vi "CliftonStrengths.vi"() -> ()   [LabVIEW 2024]
uses:
  ctrl/ctrl_white_stringBox.ctl
  ctrl/ctrl_CB_talent.ctl
  ctrl/ctrl_CB_description.ctl
  ctrl/ctrl_enum_overview.ctl
  ctrl/ctrl_enum_adj.ctl
  <vilib>/Utility/miscctls.llb/LVPointTypeDef.ctl
panel:
  out "Talent2 CB":T1
  out "arr Description CB":string[](array[string])
  out "Talent order CB":string[](array[string])
  out "Description CB":T2
  out "Talent1 CB":T1
  out "Background CB":u32(colorbox)=16777226
  out "Background black CB":u32(colorbox)
  out "comp space":u32
  out "Theme compare":string[][](array[string])=[["1 가능성을 헤아리는 능력을 타고났습니다.", "3 현실을 헤아리는 능력을 타고났습니다."], ["1 다른 여러 경로를 고려합니다.", "25 단 하나의 목적지에 집중합니다."], ["2 관심이 가면 의지도 생깁니다.", "25 의지가 있어야 관심이 생깁니다."], ["2 항상 새로운 것을 배우는 데 관심이 있습니다.", "33 항상 새로운 사람을 만나는 데 관심이 있습니다."], ["3 머리를 따릅니다.", "5 가슴을 따릅니다."], ["3 진실은 객관적이며 측정할 수 있어야 합니다.", "16 진실은 정신적인 것이며 눈에 보이지 않을 수 있습니다."], ["4 성장과 배움을 위해 탐구하는 방식으로 접근함", "17 성장과 배움을 위해 습득하는 방식으로 접근함"], ["4 이해해야 할 개념에 대해 생각함", "34 해결해야 할 문제에 대해 생각함"], ["5 다른 사람의 기분을 잘 알아맞히는 편입니다.", "6 다른 사람의 성향을 잘 알아맞히는 편입니다."], ["5 직감에 따라 무엇을 해야 할지 결정합니다.", "3 데이터를 보고 무엇을 해야 할지 결정합니다."], ["6 당신이 누구인지 압니다.", "12 당신을 알고 싶고, 당신이 나를 알아주길 원합니다."], ["6 사람에서 출발해서 그 사람에게 적절한 일을 찾습니다.", "18 일에서 출발해서 그 일에 적절한 사람을 찾습니다."], ["7 제대로 못할 거라면 아예 시작도 하지 마십시오.", "20 아무것도 안 하는 것보다 뭐라도 하는 편이 낫습니다."], ["7 일을 제대로 하지 못하면 심한 죄책감이 듭니다.", "23 성공할 기회를 놓치면 너무나 후회가 됩니다."], ["8 적극적으로 개입하여 해결하기 위해 위험을 예측합니다.", "32 위험을 피하고 최소화하기 위해 위험을 예측합니다."], ["8 확신", "2 호기심"], ["9 외부에 있는 사람들을 수용하기 위해 노력합니다.", "28 내부에 있는 사람들의 합의를 도출하기 위해 노력합니다."], ["9 한 배에 탄 모든 사람을 차별없이 받아들입니다.", "10 배에 태울 사람을 선별적으로 선택합니다."], ["10 탁월함의 기준을 충족하거나 그 이상까지 달성하고 싶습니다.", "31 최고의 자리에 오르고 싶습니다."], ["10 훌륭한 성과를 쌓아가고 싶습니다.", "34 고장난 것을 고치고 싶습니다."], ["11 다른 사람들과 이야기할 때 생각이 잘 되고 가장 많이 배웁니다.", "4 혼자서 조용히 있을 때 생각이 잘 되고 가장 많이 배웁니다."], ["11 이야기를 하는 것은 사람들에게 나의 메시지를 이해시키는 데 도움이 됩니다.", "21 역사를 다시 이야기하는 것은 사람들이 과거를 기억하는 데 도움이 됩니다."], ["12 나는 사람들에게 투명하게 속을 드러내기 때문에 아는 친구들만 초대합니다.", "9 나는 사람들을 포용하는 성향이 있어 외부 사람들도 초대합니다."], ["12 이미 알고 있는 사람들에 대해 더 자세히 알고 싶습니다.", "33 더 많은 사람들을 알고 싶습니다."], ["13 타인의 성장을 알아차리고 촉진합니다.", "10 탁월함을 알아차리고 촉진합니다."], ["13 사람이 완성되게 하는 데 관심이 있습니다.", "30 일이 완수되게 하는 데 관심이 있습니다."], ["14 발견 가능성을 높이기 위해 마음의 창을 열어 둡니다.", "25 방해 가능성을 줄이기 위해 마음의 창을 닫아 둡니다."], ["14 경쟁 우위를 차지하려면 현실에서 벗어나 창의적으로 혁신하는 접근 방식이 가장 좋습니다.", "28 경쟁 우위를 차지하려면 현실적인 관점에서 효율적으로 협업하는 접근 방식이 가장 좋습니다."], ["15 매일매일이 다른 게 좋습니다.", "27 매일매일이 똑같은 게 좋습니다."], ["15 환경의 변화에 대응합니다.", "18 환경의 변화를 유도하거나 관리합니다."], ["16 신비를 인정합니다.", "3 진실을 입증합니다."], ["16 이미 존재하고 있으나 눈에는 보이지 않는 연결된 관계를 인식합니다.", "9 종종 발생하지만 눈에는 보이지 않는 사회적 배제를 인식합니다."], ["17 유용하게 사용될 수 있는 것들을 수집하기 좋아합니다.", "2 배우는 과정이 좋습니다."], ["17 실질적인 도구를 확보해 사람들과 공유함으로써 사람들을 돕습니다.", "14 창의적인 아이디어를 구상해 사람들과 공유함으로써 사람들을 돕습니다."], ["18 다양성", "25 단일성"], ["18 여러 개의 공을 공중에서 놀리는 저글링 곡예사", "7 하나의 공만 집요하게 쫓아가는 축구 선수"], ["19 근심이 없음", "3 진지함"], ["19 칭찬은 아무리 해도 지나치지 않습니다. 그래서 나는 칭찬에 후합니다.", "32 칭찬도 지나치면 해가 됩니다. 그래서 나는 칭찬에 인색합니다."], ["20 행동을 대신할 만한 것은 없습니다.", "4 사고를 대신할 만한 것은 없습니다."], ["20 제대로 이해할 때까지 계속 행동하십시오.", "32 제대로 이해할 때 행동으로 옮기십시오."], ["21 자연스럽게 과거의 일을 기억하고 가치를 부여합니다.", "24 자연스럽게 앞으로 일어날 수 있는 일 또는 일어나야 하는 일을 예측하고 상상합니다."], ["21 과거를 이해해야 앞으로 나아갈 수 있습니다.", "25 목표가 분명해야 앞으로 나아갈 수 있습니다."], ["22 사람들을 비슷하게 대우해야 공정성이 높아집니다.", "6 사람들을 다르게 대우해야 공정성이 높아집니다."], ["22 회전목마를 좋아합니다.", "15 롤러코스터를 좋아합니다."], ["23 존경받고 싶기 때문에 존경받을 만한 일을 해야 합니다.", "33 사람들을 내 편으로 만들고 싶기 때문에 매력을 키워야 합니다."], ["23 사람들이 나를 봐주고 나의 이야기를 들어주면 좋겠습니다.", "32 내가 사람들을 지켜보고 사람들의 이야기를 들었으면 좋겠습니다."], ["24 내일에 너무 몰두한 나머지 오늘을 맞을 준비가 되어 있지 않습니다.", "15 오늘에 너무 몰두한 나머지 내일을 맞을 준비가 되어 있지 않습니다."], ["24 더 나은 세상을 볼 수 있습니다.", "1 더 나은 세상으로 가는 길을 볼 수 있습니다."], ["25 내겐 목표가 있습니다.", "24 내겐 꿈이 있습니다."], ["25 달성하려고 계획하는 목표가 있습니다.", "27 목표 달성을 위한 계획이 있습니다."], ["26 대립을 통해 상황을 명쾌하게 정리합니다.", "28 화합을 통해 합의점을 찾습니다."], ["26 사람들이 당신에게 끌리는 이유는 당신의 생각을 알기 때문입니다.", "5 사람들이 당신에게 끌리는 이유는 당신이 사람들의 감정을 잘 헤아리기 때문입니다."], ["27 마감을 지키는 이유는 기분이 좋아지기 때문입니다.", "7 마감을 지키는 이유는 그래야 사람들이 나를 존중하기 때문입니다."], ["27 나무를 보느라 숲을 보지 못합니다.", "16 숲을 보느라 나무를 보지 못합니다."], ["28 가장 잘 풀리는 일을 합시다.", "29 가장 중요한 일을 하고 싶습니다."], ["28 나는 상호의존적인 사람이라 기꺼이 전문가의 의견을 따릅니다.", "8 나는 독립적인 사람이라 나 자신의 전문성에 자신있게 의존합니다."], ["29 옳은 길은 하나뿐이므로 다른 길에는 눈길을 주지 않을 것입니다.", "1 가능한 길은 많으므로 전부 고려해 봐야 합니다."], ["29 믿는 것을 봅니다.", "3 보는 것을 믿습니다."], ["30 일을 완수하고 싶습니다.", "20 일을 시작하고 싶습니다."], ["30 치열한 성실함", "4 치열한 사고"], ["31 나는 남들의 성과를 지켜볼 때 더 나은 성과를 냅니다.", "23 나는 남들이 나의 성과를 지켜볼 때 더 나은 성과를 냅니다."], ["31 성과를 측정하는 수단이 되어 승리를 입증하는 것은 득점판입니다.", "3 경험을 수치화하고 이론을 입증하는 것은 데이터입니다."], ["32 브레이크와 같이 일의 속도를 늦추는 경향이 있습니다.", "20 가속 페달과 같이 일의 속도를 높이는 경향이 있습니다."], ["32 교제를 할 때 신중을 기함", "33 교제를 할 때 경계없이 적극적임"], ["33 넓은 인맥을 쌓을 수 있습니다.", "12 깊이 있는 인간 관계를 맺을 수 있습니다."], ["33 다른 사람을 내 편으로 만듦", "31 다른 사람을 이김"], ["34 문제 해결사", "1 지도 제작자"], ["34 의도적으로 문제 영역으로 들어가 원래 상태로 복구합니다.", "19 의도적으로 문제 영역을 피해 나의 감정 상태를 유지합니다."]]
  out "Basic info":T3(array[cluster])=[{"Talent"="", "Talent_eng"="", "Classify text"="", "설명"="", "성향"="", "행동 양상"="", "기여하는 것"="", "필요로 하는 것(요구 사항)"="", "좋아하는 것(가치)"="", "싫어하는 것(가치)"="", "은유/이미지"="", "장벽(Barrier Label)"="", "adj"="", "noun"=""}, {"Talent"="전략", "Talent_eng"="Strategic", "Classify text"="T", "설명"="일을 진행하는데 있어서 여러 가지 대안을 만듭니다. 이들은 어떠한 상황에 직면하더라도 신속하게 그 상황에 관련된 패턴과 이슈를 파악할 수 있습니다.", "성향"="최상의 기회를 놓치지 않도록 모든 가능성을 고려하려는 의지가 있음", "행동 양상"="앞으로 나아갈 최선의 길을 찾음", "기여하는 것"="창의적인 예측, 상상력, 끈기", "필요로 하는 것(요구 사항)"="도중에 경로를 수정할 수 있는 재량", "좋아하는 것(가치)"="방법이 없다는 사람들의 판단에도 불구하고 방법을 찾는 것", "싫어하는 것(가치)"="늘 하던 대로 일을 처리하는 것", "은유/이미지"="넓은 주변 시야 - 전체를 볼 수 있음", "장벽(Barrier Label)"="항상 다른 것을 시도해야 함", "adj"="창의적인\n분명한\n옵션을 생각하는\n직관적인\n미래지향적인\n예상을 하는\n선별적인\n사려 깊은\n통찰력 있는", "noun"="선택하는 사람\n사색가\n전략가\n선별자\n분류자\n평가자\n지도 제작자\n길을 찾는 사람\n계획가"}, {"Talent"="배움", "Talent_eng"="Learner", "Classify text"="T", "설명"="배움에 대한 강한 열망이 있으며, 끊임없이 발전하고 싶어 합니다. 배움의 결과물보다는 배우는 과정 자체가 이들을 신나게 합니다.", "성향"="배우는 과정을 즐김", "행동 양상"="흥미를 불러일으키는 것들에 대해 알아보려고 함", "기여하는 것"="배움의 관점과 배우는 과정에 대한 열정", "필요로 하는 것(요구 사항)"="새로운 정보와 경험을 접하는 것", "좋아하는 것(가치)"="새로운 분야, 최첨단을 계속 익히는 것", "싫어하는 것(가치)"="뭐든지 다 아는 척, 똑똑한 척하는 것", "은유/이미지"="지속적인 배움은 Yes, 배움의 정체는 No", "장벽(Barrier Label)"="호기심으로 인해 불필요한 결과를 초래하거나 생산성을 떨어뜨릴 수 있음", "adj"="호기심이 많은\n흥미가 있는\n탐구심이 많은\n개방적인\n학구적인\n열성적인\n역량이 있는", "noun"="학생\n탐험가\n발견자\n스스로 돕는 사람\n꾸준히 성장하는 사람\n전문가"}, {"Talent"="분석", "Talent_eng"="Analytical", "Classify text"="T", "설명"="이유와 원인을 찾습니다. 이들에게는 특정한 상황에 영향을 미칠 수 있는 모든 요인에 대해 생각하는 능력이 있습니다.", "성향"="접근 방식이 논리적이고 객관적임", "행동 양상"="복잡성 속에서 단순함을 발견함", "기여하는 것"="감정적인 이슈에 대한 냉철한 사고", "필요로 하는 것(요구 사항)"="생각할 시간", "좋아하는 것(가치)"="자료와 사실", "싫어하는 것(가치)"="입증되지 않거나 입증할 수 없는 것들", "은유/이미지"="불필요한 요소를 없애고 핵심만 남김", "장벽(Barrier Label)"="분석에 치중하느라 아무것도 하지 못함", "adj"="객관적인\n숫자를 중시하는\n데이터를 근거로 하는\n냉정한\n회의적인\n호기심 많은\n과학적인", "noun"="과학자\n측정가\n계산하는 사람\n팩트 탐색자/사용자\n관찰자\n논리에 능한 사람"}, {"Talent"="지적사고", "Talent_eng"="Intellection", "Classify text"="T", "설명"="지적인 활동을 하는 특징이 있습니다. 이들은 자기 성찰적이며 지적인 토론을 즐깁니다.", "성향"="개념에 대해 생각하고, 심오하며, 혼자 있기를 좋아함", "행동 양상"="사고와 실행이 다를 바 없다고 생각함", "기여하는 것"="깊이 있는 이해와 지혜", "필요로 하는 것(요구 사항)"="성찰과 명상을 위한 시간", "좋아하는 것(가치)"="이론. 실질적인 것이 탄생하는 밑거름이므로", "싫어하는 것(가치)"="매사에 생각 없이 접근하는 태도", "은유/이미지"="깊이 파헤치는 모습", "장벽(Barrier Label)"="고립되어 있고 거리를 둠", "adj"="자기 성찰적인\n혼자서 잘 지내는\n지적인\n철학적인\n깊이가 있는\n사색적인\n만족하지 않는\n생각에 잠기는\n강렬한\n깊이 생각하는\n의욕이 넘치는", "noun"="생각하는 사람\n철학자\n토론자\n명상가\n혼자 있기를 좋아하는 사람\n작가\n블로거"}, {"Talent"="공감", "Talent_eng"="Empathy", "Classify text"="R", "설명"="자신이 다른 사람의 삶이나 상황 속에 있는 것처럼 상상함으로써 다른 사람의 감정을 느낄 수 있습니다.", "성향"="감성적임", "행동 양상"="감정을 명확하게 표현함", "기여하는 것"="감성지능(emotional intelligence)", "필요로 하는 것(요구 사항)"="웃고 울고 감정을 발산할 자유", "좋아하는 것(가치)"="인간의 희로애락", "싫어하는 것(가치)"="감정 표현을 차단하거나 제한하는 것들", "은유/이미지"="개인적 감정이 결정에 영향을 미치는 일이 자주 있음", "장벽(Barrier Label)"="동정심이 지나침", "adj"="경청하는\n감성적인\n표현을 잘하는\n섬세한\n알아차리는\n직관적인\n비밀을 지키는\n도움을 주는\n감각적인", "noun"="감정을 느끼는 사람\n비밀을 지키는 친구\n표현을 잘하는 사람\n현명한 사람\n받아들이는 사람\n경청하는 사람\n공감하는 사람"}, {"Talent"="개별화", "Talent_eng"="Individualization", "Classify text"="R", "설명"="각 사람이 지닌 독특한 개성에 흥미를 느낍니다. 이들은 서로 달느 사람들이 어떻게 협력하여 생산적으로 일할 수 있는지 파악하는 데 재능이 있습니다.", "성향"="상황을 각 개인에 맞춰줌", "행동 양상"="인간의 다양성이 지닌 문제점보다는 잠재력에 주목함", "기여하는 것"="사람을 잘 이해하여 인력 배치에 도움을 줌", "필요로 하는 것(요구 사항)"="개인 맞춤형 기대치 설정", "좋아하는 것(가치)"="사람들이 각자 가장 잘하는 일을 하게 되는 것", "싫어하는 것(가치)"="한 가지 방식을 모든 상황에 적용하는 접근 방식", "은유/이미지"="배역 담당자 - 배우들에 대해 알고 있는 사항을 활용함", "장벽(Barrier Label)"="개인의 요구를 충족하기 위해 집단의 요구를 희생함", "adj"="알아차리는\n독특한\n직관력이 있는\n사람을 중시하는\n강점을 중시하는\n기민한\n공정한\n정확한\n통찰력이 있는\n다양성을 중시하는", "noun"="개인화하는 사람\n관찰자\n받아들이는 사람\n알아차리는 사람\n물색하는 사람\n인류학자\n소설가\n전기 작가"}, {"Talent"="책임", "Talent_eng"="Responsibility", "Classify text"="E", "설명"="자신이 하겠다고 약속한 것들에 대해서 강한 주인의식(ownership)을 느낍니다. 이들은 정직성과 충실함 같은 가치관을 매우 중요시 합니다.", "성향"="일을 완수하리라 믿고 맡길 수 있는 사람임", "행동 양상"="약속을 최선을 다해 끝까지 지킴", "기여하는 것"="신뢰와 충실함", "필요로 하는 것(요구 사항)"="주인 의식을 가질 수 있는 재량", "좋아하는 것(가치)"="다른 사람들의 존경", "싫어하는 것(가치)"="사람들을 실망시키고 사람들에게 실망하는 것", "은유/이미지"="무관심한 세입자가 아닌 진지한 소유주", "장벽(Barrier Label)"="거절하지 못하고, 쉽게 놓지 못함", "adj"="근면한\n양심적인\n판단을 하는\n충성스러운\n의욕적인\n임무를 완수하는\n믿음직스러운\n진지한\n헌신적인\n자기 희생적인\n즉각 반응하는\n독립적인", "noun"="주인의식이 있는 사람\n노력하는 사람\n섬김의 정신이 강한 사람\n응답하는 사람\n완벽주의자\n심판\n자원자\n제어하는 사람"}, {"Talent"="자기확신", "Talent_eng"="Self-Assurance", "Classify text"="I", "설명"="위험을 감수하고 삶을 이끌어가는 자신의 능력에 대한 자신감을 가지고 있습니다. 이들에게는 자신의 의사결정에 확신을 갖게 하는 내면의 나침반이 있습니다.", "성향"="외부적으로 불확실한 상황에서도 자신감을 유지함", "행동 양상"="영향을 받기보다 영향력을 행사하고자 함", "기여하는 것"="필요한 위험을 감수할 의지", "필요로 하는 것(요구 사항)"="일방적, 독립적으로 활동할 수 있는 재량", "좋아하는 것(가치)"="운명은 스스로 결정하는 것이라는 태도", "싫어하는 것(가치)"="다른 사람의 지시", "은유/이미지"="마음의 나침반, 내면의 북소리에 맞춰 행진하는 모습", "장벽(Barrier Label)"="오만, 지나친 자신감, 자기 만족", "adj"="독립적인\n확신하는\n자신감 있는\n자의식 있는\n자립적인\n본능적인\n강렬한\n통제하는\n안정적인\n집요한", "noun"="인플루엔서\n통제자\n감독\n위험 감수자\n리더"}, {"Talent"="포용", "Talent_eng"="Includer", "Classify text"="R", "설명"="다른 사람을 받아들입니다. 이들은 소외되었다고 느끼는 사람을 알아차리고 그들을 포용하기 위해 노력합니다.", "성향"="배제된 사람을 알아차리고 그로 인해 초래될 영향을 이해함", "행동 양상"="가진 자와 못 가진 자의 격차를 줄임", "기여하는 것"="다양성 수용에 대한 높은 수준의 관용", "필요로 하는 것(요구 사항)"="누구나 받아들일 수 있는 여지", "좋아하는 것(가치)"="동화와 통합", "싫어하는 것(가치)"="패거리 문화", "은유/이미지"="모토 - 여기서는 누구나 환영합니다", "장벽(Barrier Label)"="무분별함", "adj"="기꺼이 받아들이는\n인내심이 있는\n상호적인\n직관력이 있는\n타인 지향적인\n반갑게 맞이하는\n세심한\n통합하는", "noun"="수용가\n용인하는 사람\n초청자\n환영하는 사람\n동화시키는 사람\n장벽을 허무는 사람"}, {"Talent"="최상화", "Talent_eng"="Maximizer", "Classify text"="I", "설명"="개인이나 집단의 탁월성을 자극하기 위해 그들의 강점에 초점을 맞춥니다. 이들은 좋은 것을 최상의 것으로 전환시킬 방법을 찾습니다.", "성향"="탁월성을 이끌어내는 데 전념함", "행동 양상"="강점에 집중하면서 약점을 관리함", "기여하는 것"="품질 지향", "필요로 하는 것(요구 사항)"="양만큼 질도 중시되어야 함", "좋아하는 것(가치)"="최대의 ROI(Return on Investment, 투자 대비 수익)", "싫어하는 것(가치)"="약점을 고치려는 집착", "은유/이미지"="'좋음'에서 '탁월함'으로, Good-Better-Best", "장벽(Barrier Label)"="까다롭고 만족을 모름", "adj"="선별적인\n강점을 중시하는\n품질을 중시하는\n결과를 중시하는\n강점에 매료되는\n탁월함을 의식하는\n까다로운\n판단을 하는\n가려내는\n만족하지 않는", "noun"="리더\n추진가\n명확하게 밝히는 사람\n설득자\n파이터\n도전자\n요구가 많은 사람\n완벽주의자\n품질 관리자"}, {"Talent"="커뮤니케이션", "Talent_eng"="Communication", "Classify text"="I", "설명"="대체로 쉽게 자신의 생각을 말로 표현합니다. 이들은 대화와 발표에 능합니다.", "성향"="말솜씨가 있음", "행동 양상"="말을 통해 타인과 관계를 구축함", "기여하는 것"="사람들이 들어야 할 메시지에 주의를 집중시킴", "필요로 하는 것(요구 사항)"="반응해주는 사람들, 청중", "좋아하는 것(가치)"="이야기와 이야기꾼", "싫어하는 것(가치)"="표현하지 못한 경험", "은유/이미지"="침묵은 금이 아님", "장벽(Barrier Label)"="수다스러움", "adj"="말하기 좋아하는\n발표를 잘하는\n언어 능력이 있는\n투명한\n상호적인\n대화에 능한\n표현력이 뛰어난\n사로잡는\n재미있는", "noun"="말하는 사람\n발표자\n대화에 능한 사람\n스토리텔러\n말솜씨가 좋은 사람\n설명하는 사람\n작가"}, {"Talent"="절친", "Talent_eng"="Relator", "Classify text"="R", "설명"="주변 사람들과 깊고 친밀한 관계를 맺는 것을 좋아합니다. 이들은 친밀한 사람들과 함께 목표를 향해 열심히 일하는 데에서 깊은 만족감을 얻습니다.", "성향"="진실되고 믿음직스러움", "행동 양상"="가까운 사람들에 대해 더 많이 알아감", "기여하는 것"="깊이 있고 투명한 대인관계", "필요로 하는 것(요구 사항)"="사람들과 일대일 교류할 수 있는 시간과 기회", "좋아하는 것(가치)"="서로를 챙겨주는 친밀한 상호 관계", "싫어하는 것(가치)"="새로운 사람을 처음 만났을 때의 불편함", "은유/이미지"="서로를 잘 아는 친구", "장벽(Barrier Label)"="파벌에 따른, 정에 이끌린 인사를 함", "adj"="친절한\n배려심 있는\n진정성 있는\n진실된\n친밀한\n투명한\n정직한\n자신을 드러내는", "noun"="친구\n가족\n충직한 사람\n다른 사람을 돌보는 사람"}, {"Talent"="개발", "Talent_eng"="Developer", "Classify text"="R", "설명"="다른 사람의 잠재력을 알아보고 이를 키워줍니다. 이들은 작은 진전의 신호를 알아차리며 사람들이 발전해가는 모습에서 만족을 얻습니다.", "성향"="경험이 부족하고 미숙한 사람들에 대해 인내심이 있음", "행동 양상"="타인의 성장에서 만족감을 느낌", "기여하는 것"="사람의 성장에 헌신할 시간과 에너지", "필요로 하는 것(요구 사항)"="투자할 대상자", "좋아하는 것(가치)"="인간의 잠재력과 진보", "싫어하는 것(가치)"="잠재력이 낭비되거나 실현되지 않는 것", "은유/이미지"="걸음마를 배우는 아기를 인내하며 지켜보는 부모", "장벽(Barrier Label)"="저성과자에게 시간을 낭비함", "adj"="참을성이 있는\n직관력이 있는\n유능한\n격려를 잘하는\n시간과 노력을 투자하는\n타인 지향적인\n관찰력이 있는\n성장을 중시하는\n자기 희생적인\n다른 사람에게 도움을 주는", "noun"="투자자\n코치\n멘토\n교사\n격려하는 사람\n역량을 개발해주는 사람"}, {"Talent"="발상", "Talent_eng"="Ideation", "Classify text"="T", "설명"="아이디어에 매료됩니다. 이들은 보기에는 상관없어 보이는 현상들의 연관성을 찾아낼 수 있습니다.", "성향"="혁신에 내포된 애매모호함과 위험 요소에 영향을 받지 않음", "행동 양상"="고정관념에서 벗어난 사고를 함", "기여하는 것"="새롭고 신선한 시각", "필요로 하는 것(요구 사항)"="통제나 제한없이 가능성을 탐색할 자유", "좋아하는 것(가치)"="완전히 새로운 무엇인가를 제시하는 것", "싫어하는 것(가치)"="늘 하던 일을 하는 것", "은유/이미지"="예술가의 창의력, 비어 있는 캔버스나 백지, 찰흙", "장벽(Barrier Label)"="비현실적임", "adj"="즉흥적인\n창의적인\n혁신적인\n예술적인\n통찰력이 있는\n지략이 풍부한\n활기를 주는", "noun"="발명가\n창조자\n디자이너\n예술가\n혁신자\n브레인스토머\n소설가"}, {"Talent"="적응", "Talent_eng"="Adaptability", "Classify text"="R", "설명"="상황의 흐름에 따라 적응하는 것을 선호합니다. 이들은 일이 생기는 대로 받아들이며 미래에 대해서는 그때 가서 대처하려 하며, '현재'에 충실한 경향이 있습니다.", "성향"="\"지금 바로 여기\"를 중시함", "행동 양상"="당면한 상황에 즉각적으로 대응함", "기여하는 것"="변화가 일어나는 방향으로 기꺼이 따라감", "필요로 하는 것(요구 사항)"="즉각적 대응을 필요로 하는 현재의 압력", "좋아하는 것(가치)"="즉흥성", "싫어하는 것(가치)"="예측 가능성", "은유/이미지"="강물처럼 흐름에 따라감", "장벽(Barrier Label)"="방향성이 없음", "adj"="유연한\n먼저 반응하는\n느긋한\n현재에 집중하는\n순간에 충실한\n즉흥적인\n선뜻 동의하는\n실존주의적인", "noun"="먼저 반응하는 사람\n얼리 어답터\n적응하는 사람\n추종자"}, {"Talent"="연결성", "Talent_eng"="Connectedness", "Classify text"="R", "설명"="모든 것들이 연결되어 있다고 믿습니다. 이들은 우연이란 거의 존재하지 않으며 일어나는 거의 모든 일에는 다 의미가 있다고 믿습니다.", "성향"="인류는 국경과 시간을 초월하는 하나의 가족이라고 생각함", "행동 양상"="부분을 전체로 통합함", "기여하는 것"="생명과 모든 우주 만물의 신비와 경이를 인지하고 감사함", "필요로 하는 것(요구 사항)"="자신보다 더 큰 무언가(가족, 팀, 글로벌 커뮤니티, 우주 등)의 일부가 되는 것", "좋아하는 것(가치)"="삶의 순환, 연결의 끈", "싫어하는 것(가치)"="\"편 가르기\" 사고방식", "은유/이미지"="몸, 마음, 영혼이 연결된 사람", "장벽(Barrier Label)"="괴짜, 뉴에이지 애호가, 현실과 동떨어짐", "adj"="통합하는\n탐구하는\n영적인\n위안을 주는\n직관력이 있는\n신비로운\n철학적인\n상담을 해주는\n경청하는", "noun"="통합가\n다리가 되어 주는 사람\n환경주의자\n인도주의자\n공동체주의자\n통합하는 사람\n사회운동가\n탐구자"}, {"Talent"="수집", "Talent_eng"="Input", "Classify text"="T", "설명"="수집하고 보관하고 싶어합니다. 이들은 정보, 아이디어, 작품이나 심지어 관계도 축적할 수 있습니다.", "성향"="실용적인 자원 수집가", "행동 양상"="다른 사람들에게 유용한 자원이 될 수 있는 것들을 수집함", "기여하는 것"="성장과 성과를 촉진할 수 있는 구체적인 도구", "필요로 하는 것(요구 사항)"="자연스럽게 수집하게 된 자원을 보관할 공간", "좋아하는 것(가치)"="관련성이 높은 실질적인 도움을 제공하는 것", "싫어하는 것(가치)"="다른 사람들에게 유용할 만한 자원을 확보하지 못하는 것", "은유/이미지"="흡수(input)하고 내보내는(output) 스펀지", "장벽(Barrier Label)"="필요도 없는 잡다한 것들을 되는대로 쌓아놓음", "adj"="지략이 풍부한\n수집을 즐기는\n탐구심이 많은\n관대한\n박식한\n정통한\n조사에 능한", "noun"="보관하는 사람\n도서관 사서\n수집가\n흡수하는 사람\n큐레이터\n자원을 수집하는 사람\n전달자"}, {"Talent"="정리", "Talent_eng"="Arranger", "Classify text"="E", "설명"="복잡한 상황을 체계적으로 정리할 수 있는 능력과 함께 이를 보완해주는 유연성도 가지고 있습니다. 이들은 생산성을 최대화하기 위해 모든 구성요소와 자원을 최적으로 정리하는 것을 좋아합니다.", "성향"="변수가 많아도 편안함", "행동 양상"="다른 사람들을 통해 더 효과적이고 효율적으로 업무를 수행함", "기여하는 것"="유연성과 상호작용", "필요로 하는 것(요구 사항)"="역동적인 환경", "좋아하는 것(가치)"="필요한 변화의 시작과 관리", "싫어하는 것(가치)"="필요한 변화에 대한 저항", "은유/이미지"="지휘자, 코디네이터", "장벽(Barrier Label)"="너무 잦은 변경으로 쫓아가기 어려움", "adj"="유연한\n상호적인\n통제를 잘하는\n협력적인\n동시에 여러 가지를 고려하는\n구성에 능한\n즉각적인\n지략이 풍부한", "noun"="저글러\n조율가\n코디네이터\n재배열하는 사람\n멀티 씽커(Multi thinker)\n통제자\n협력자\n지휘자"}, {"Talent"="긍정", "Talent_eng"="Positivity", "Classify text"="R", "설명"="주변 사람들을 쉽게 사로잡는 긍정적인 열정을 가지고 있습니다. 이들은 낙관적이며 사람들로 하여금 자신들이 하려는 일에 열의를 갖게 만듭니다.", "성향"="낙관적이고 희망적이며 재미를 추구함", "행동 양상"="사기를 북돋는 밝은 정서적 환경을 조성함", "기여하는 것"="전염성이 강한 힘과 열정", "필요로 하는 것(요구 사항)"="삶의 기쁨과 극적인 순간을 경험할 자유", "좋아하는 것(가치)"="삶을 충만하게 영위", "싫어하는 것(가치)"="다른 사람을 기운 빠지게 하는 부정적인 사람들", "은유/이미지"="절반밖에 안 남은 유리잔이 아닌 절반이나 차있는 유리잔", "장벽(Barrier Label)"="너무 순진함", "adj"="재미있는\n낙관적인\n희망을 주는\n관대한\n들떠 있는\n행복한\n열광적인\n힘이 넘치는\n기쁨을 주는\n영향적이 있는\n호들갑스러운\n걱정이 없는\n긍정적인", "noun"="에너자이저\n낙관주의자\n격려자\n영향력을 미치는 사람\n코미디언\n예능인\n축하하는 사람\n인정하는 사람\n열렬한 지지자\n옹호자\n"}, {"Talent"="행동", "Talent_eng"="Activator", "Classify text"="I", "설명"="머리 속에 있는 생각을 행동으로 옮겨 실현시킬 수 있습니다. 이들은 말만 하기 보다는 당장 실행하기를 원합니다.", "성향"="아무것도 안 하는 상황을 참을 수 없음", "행동 양상"="추진력을 만들어냄", "기여하는 것"="긴박함을 불어넣음", "필요로 하는 것(요구 사항)"="토론은 적게, 행동은 많이", "좋아하는 것(가치)"="시작, 착수", "싫어하는 것(가치)"="기다림, 시간 낭비", "은유/이미지"="빠른 착수", "장벽(Barrier Label)"="두들겨보기도 전에 돌다리를 건넘", "adj"="참을성 없는\n영향력 있는\n행동 지향적인\n주도적인\n촉매제 역할을 하는\n추진력이 있는\n빠른", "noun"="촉매제\n주도적인 사람\n선동자\n착수자\n인플루엔서"}, {"Talent"="회고", "Talent_eng"="Context", "Classify text"="T", "설명"="과거에 대해서 생각하는 것을 즐깁니다. 이들은 과거에 대한 성찰을 통해서 현재를 이해합니다.", "성향"="조상을 감사히 여기고 과거 사건들을 중요하게 여김", "행동 양상"="중요한 역사를 기억함", "기여하는 것"="정확한 기억과 귀중한 수집품", "필요로 하는 것(요구 사항)"="논의를 진행하고 결정을 내리기 위한 관련 배경", "좋아하는 것(가치)"="회고", "싫어하는 것(가치)"="과거에 대한 망각", "은유/이미지"="백미러 - 안전 운전을 위한 필수 요소", "장벽(Barrier Label)"="과거에서 벗어나지 못함", "adj"="역사에 관심이 높은\n과거를 중시하는\n직관력이 있는\n강조하는\n수집을 즐기는\n학구적인", "noun"="역사가\n프레임제시자\n기록자\n고고학자\n족보학자"}, {"Talent"="공정성", "Talent_eng"="Consistency", "Classify text"="E", "설명"="사람들이 동등하게 취급되어야 한다는 점을 날카롭게 인식합니다. 이들은 모두가 따를 수 있는 안정적인 루틴과 명료한 규칙, 절차를 갈망합니다.", "성향"="개인이 무엇을 바라는지보다 그룹이 무엇을 필요로 하는지에 더 많은 관심을 가짐", "행동 양상"="차이를 줄이고 균일성을 높임", "기여하는 것"="예측 가능한 문화를 조성하는 규칙과 정책", "필요로 하는 것(요구 사항)"="표준적인 운영 절차", "좋아하는 것(가치)"="동일한 방식으로 무엇인가를 반복하는 것", "싫어하는 것(가치)"="불필요한 맞춤화", "은유/이미지"="대열을 맞춰 비행하는 한무리의 거위 떼", "장벽(Barrier Label)"="관계와 결과보다 규칙을 우선시함", "adj"="공정한\n똑같이 하는\n평등하게 대하는\n원칙적인\n예측 가능한\n일관성 있는\n정당한\n현실적인\n효율적인", "noun"="표준화하는 사람\n규칙 집행자\n체계를 만드는 사람\n심판"}, {"Talent"="존재감", "Talent_eng"="Significance", "Classify text"="I", "설명"="큰 영향을 미치기를 원합니다. 그들은 독립적이며, 프로젝트의 우선순위를 정할 때 그것이 조직이나 주위 사람들에게 얼마나 영향을 미칠지를 근거로 생각합니다.", "성향"="사람들에게 중요한 존재로 인식되어 중요한 일을 맡아 완수할 수 있는 기회에 관심이 있음", "행동 양상"="다른 사람들의 인식에서 영향을 받고 이를 통해 의욕을 냄", "기여하는 것"="더 많이 인정받고 싶어하는 마음", "필요로 하는 것(요구 사항)"="기량을 최대로 발휘할 의욕을 갖게 하고, 나의 진가를 알아봐 주는 사람들", "좋아하는 것(가치)"="성공한 사람들과의 교류", "싫어하는 것(가치)"="다른 사람들에게 존재감이 없거나 무시 당하는 것", "은유/이미지"="무대 중앙에 서거나 조명을 받는 것을 편하게 여기는 타고난 연예인", "장벽(Barrier Label)"="주목 받을 일만을 찾아 다님, 과시적임", "adj"="존경 받는\n믿을 수 있는\n성공적인\n눈에 띄는\n영향력이 있는\n원하는 것이 있는\n독립적인\n청중을 의식하는\n전문적인\n특출난", "noun"="손을 뻗는 사람\n예능인\n스타\n추구하는 사람\n열망하는 사람\n갈망하는 사람\n욕망하는 사람\n주장하는 사람"}, {"Talent"="미래지향", "Talent_eng"="Futuristic", "Classify text"="T", "설명"="미래와 가능성에서 영감을 얻습니다. 이들은 미래의 비전으로 사람들에게 영감을 줍니다.", "성향"="미래에 매료됨", "행동 양상"="앞으로 일어날 수 있는 일 또는 일어나야 하는 일을 예측하고 상상함", "기여하는 것"="미리 그려보기, 예상, 예측", "필요로 하는 것(요구 사항)"="예견되는 미래에 대해 말할 기회", "좋아하는 것(가치)"="미래를 생각하는 과정에서 얻는 영감", "싫어하는 것(가치)"="현재 상황에 만족하는 안일함", "은유/이미지"="비전", "장벽(Barrier Label)"="뜬구름 잡기", "adj"="창의적인\n영감을 주는\n상상력이 뛰어난\n상상력이 풍부한\n예상을 잘하는\n표현력이 뛰어난\n의사소통 능력이 있는\n직관력이 있는\n미래 지향적인", "noun"="예측가\n비전가\n꿈꾸는 사람\n앞을 내다보는 사람\n상상하는 사람\n예상하는 사람"}, {"Talent"="집중", "Talent_eng"="Focus", "Classify text"="E", "설명"="방향을 정해 일을 완수하며, 방향에서 벗어나지 않기 위해 필요한 수정을 해냅니다. 이들은 우선순위를 정한 다음, 실행합니다.", "성향"="굉장히 고지식하며 일부러 그런 태도를 고집함", "행동 양상"="목표에 도달할 때까지 인내함", "기여하는 것"="집중과 방향을 통한 명료함", "필요로 하는 것(요구 사항)"="우선순위를 설정할 수 있게 해주는 목표", "좋아하는 것(가치)"="끝을 염두에 둔 시작", "싫어하는 것(가치)"="잘못된 옆길로 새는 것", "은유/이미지"="무아지경", "장벽(Barrier Label)"="목적지에 도달하는 데 정신이 집중되어 있어 여정의 즐거움을 느끼지 못할 수 있음", "adj"="목표 지향적인\n끈기 있는\n의욕이 넘치는\n효율적인\n전념을 다하는\n진전을 중시하는\n선별적인\n집중을 방해하는 것을 피하는", "noun"="집중하는 사람\n우선순위를 정하는 사람\n방향을 잡는 사람\n목표를 설정하는 사람\n감독\n가이드"}, {"Talent"="주도력", "Talent_eng"="Command", "Classify text"="I", "설명"="존재감이 있습니다. 이들은 상황을 주도하고 의사결정을 내릴 수 있습니다.", "성향"="단도직입적이며 결단력이 있음", "행동 양상"="압력이 들어오면 저항함", "기여하는 것"="명확한 감정", "필요로 하는 것(요구 사항)"="도전과 갈등", "좋아하는 것(가치)"="통제를 벗어난 듯한 상황에서 통제력을 행사하는 것", "싫어하는 것(가치)"="소극적이고 회피하는 태도", "은유/이미지"="운전대를 잡고 있어야 편안함을 느낌", "장벽(Barrier Label)"="우두머리, 독재자", "adj"="결단력이 있는\n명확하게 하는\n의욕이 넘치는\n설득력 있는\n도전적인\n위압감을 주는\n단정적인\n통제적인\n자기 주장이 강한\n강요하는\n확고한\n솔직한", "noun"="통제가\n리더\n주도자\n명확하게 하는 사람\n설득자\n파이터\n도전자\n위압감을 주는 사람"}, {"Talent"="체계", "Talent_eng"="Discipline", "Classify text"="E", "설명"="정해진 절차와 구조를 즐깁니다. 스스로 만든 질서가 이들이 사는 세계를 가장 잘 설명해줍니다.", "성향"="제한된 자원을 효율적으로 관리함", "행동 양상"="미리 계획하고 그 다음에 계획을 따름", "기여하는 것"="정확성과 세부 지향", "필요로 하는 것(요구 사항)"="구조화되고 질서 있는 환경", "좋아하는 것(가치)"="질서 정연하게 정리된 것", "싫어하는 것(가치)"="혼란, 혼동, 감으로 일하는 것", "은유/이미지"="일렬로 줄지어가는 오리떼", "장벽(Barrier Label)"="변화에 저항할 수 있음", "adj"="예측 가능한\n세심한\n조직적인\n효율적인\n꼼곰한\n구조적인\n깔끔한\n정돈된\n시기적절한\n예행연습을 하는\n계획적인\n정확한", "noun"="조직가\n계획가\n자율통제자\n설계자\n구성하는 사람\n완벽주의자"}, {"Talent"="화합", "Talent_eng"="Harmony", "Classify text"="R", "설명"="합의를 추구합니다. 이들은 갈등을 좋아하지 않고 갈등 대신 합의점을 찾고자 합니다.", "성향"="침착하고 평온함", "행동 양상"="감정적 에너지 소모를 없애려고 노력함", "기여하는 것"="평화와 사랑, 갈등을 피하는 접근법", "필요로 하는 것(요구 사항)"="합의점, 공통된 의견", "좋아하는 것(가치)"="그룹의 성과를 높이기 위해 개인적 주장을 희생함", "싫어하는 것(가치)"="갈등으로 인한 부정적 영향", "은유/이미지"="불편한 마음을 달램", "장벽(Barrier Label)"="갈등을 두려워함", "adj"="현실적인\n구체적인\n갈등을 줄이는\n협력적인\n선뜻 동의하는\n과업지향적인", "noun"="현실주의자\n실용주의자\n평화주의자\n협상가\n중재자\n대사\n외교관"}, {"Talent"="신념", "Talent_eng"="Belief", "Classify text"="E", "설명"="변하지 않는 확고한 핵심 가치를 가지고 있습니다. 이들의 삶의 목적은 이러한 가치에서 나옵니다.", "성향"="핵심 가치에 대한 열정이 있으며, 이를 타협하지 않음", "행동 양상"="중요한 일을 위해 기꺼이 희생함", "기여하는 것"="안정성, 명확성, 신념을 중시함", "필요로 하는 것(요구 사항)"="삶의 이유 또는 목적", "좋아하는 것(가치)"="이타심", "싫어하는 것(가치)"="신념에 맞지 않는 모든 것", "은유/이미지"="믿음을 전파하는 선교사", "장벽(Barrier Label)"="고집불통임", "adj"="확신이 있는\n안정적인\n변함없는\n지조있는\n열성적인\n헌신적인\n자기 희생적인", "noun"="선교사\n기여자\n믿는 사람\n이타주의자"}, {"Talent"="성취", "Talent_eng"="Achiever", "Classify text"="E", "설명"="에너지가 왕성하며 열심히 일합니다. 이들은 바쁘고 생산적인 데서 큰 만족감을 얻습니다.", "성향"="열심히 일함", "행동 양상"="업무 속도를 주도적으로 정함", "기여하는 것"="강도 높고 지치지 않는 노력", "필요로 하는 것(요구 사항)"="자신의 속도대로 일하는 재량권", "좋아하는 것(가치)"="업무 완수", "싫어하는 것(가치)"="성실하지 않은 태도", "은유/이미지"="경주 완주, 결승점 도착", "장벽(Barrier Label)"="사람보다 일을 더 중요하게 생각함", "adj"="의욕이 넘치는\n부지런한\n강렬한\n스스로 동기가 높은\n생산적인\n야심 있는\n독립적인", "noun"="수행자\n작업자\n생산자\n실행하는 사람\n마무리 짓는 사람\n완성가"}, {"Talent"="승부", "Talent_eng"="Competition", "Classify text"="I", "설명"="자신의 진전을 다른 사람의 성과와 비교해서 평가합니다. 이들은 1등을 차지하기 위해 분투하며 경쟁을 즐깁니다.", "성향"="경쟁자를 의식함", "행동 양상"="이기려고 노력함", "기여하는 것"="최고가 되려는 포부", "필요로 하는 것(요구 사항)"="비교 대상 및 동기부여가 되는 동료", "좋아하는 것(가치)"="최고의 자리에 있는 사람과 맞설 기회", "싫어하는 것(가치)"="2등을 하는 것", "은유/이미지"="아차상은 의미가 없으며 금메달만 인정함", "장벽(Barrier Label)"="패배를 인정하지 않음", "adj"="점수를 기록하는\n비교하는\n승리하는\n측정하는\n포부가 큰\n의욕이 넘치는\n강렬한\n선별적인", "noun"="승자\n점수 기록자\n비교하는 사람\n측정가"}, {"Talent"="심사숙고", "Talent_eng"="Deliberative", "Classify text"="E", "설명"="의사결정을 하거나 선택할 때 매우 신중합니다. 이들은 장애요소를 예측합니다.", "성향"="잠재적 위험을 관찰하는 데 경계를 늦추지 않음", "행동 양상"="잘못될 가능성이 있는 일을 예측함", "기여하는 것"="철저하고 성실한 접근", "필요로 하는 것(요구 사항)"="의견을 내기 전에 듣고 생각할 시간", "좋아하는 것(가치)"="리스크 직면 시 통제와 주의", "싫어하는 것(가치)"="성급한 판단", "은유/이미지"="유비무환, 평결에 앞서 숙고 과정을 거치는 배심원", "장벽(Barrier Label)"="망설임 - 아침에 일찍 일어나는 새가 벌레를 잡음에도 불구하고", "adj"="주의 깊은\n신중한\n보수적인\n분별 있는\n사려 깊은\n진지한\n비밀을 지키는\n관찰력이 있는\n방심하지 않는\n위험을 무릎쓰지 않는\n남에게 자기 얘기를 잘 안하는\n원칙을 따르는", "noun"="위험을 가늠하는 사람\n예방하는 사람\n수호자\n계획하는 사람"}, {"Talent"="사교성", "Talent_eng"="Woo", "Classify text"="I", "설명"="새로운 이들을 만나 그들의 마음을 얻는 일에 도전하기를 무척 즐깁니다. 이들은 어색한 분위기를 깨고 다른 사람과 인맥을 쌓는 데에서 만족감을 얻습니다.", "성향"="사람들과 금방 친해지고 외향적임", "행동 양상"="사람들과 교제할 때 주도권을 잡음", "기여하는 것"="사람들이 모이는 자리에 활기를 불어넣음", "필요로 하는 것(요구 사항)"="다양한 사람들과의 만남", "좋아하는 것(가치)"="처음 보는 사람과의 만남", "싫어하는 것(가치)"="정체되거나 위축된 인맥", "은유/이미지"="아이스 브레이킹 - 먼저 악수를 청함", "장벽(Barrier Label)"="겉치레를 중시하고 가벼움", "adj"="매력적인\n상호적인\n사회성이 강한\n영향력이 있는\n외향적인\n사교적인\n끌어들이는\n주도적인\n마음을 끄는\n사교적 에너지가 넘치는", "noun"="사교적인 사람\n매력적인 사람\n대화에 능한 사람\n접대자\n관계를 잘 맺는 사람\n먼저 시작하는 사람\n네트워커\n탐사자"}, {"Talent"="복구", "Talent_eng"="Restorative", "Classify text"="E", "설명"="문제를 능숙하게 다룹니다. 이들은 무엇이 잘못되었는지 파악하고 이를 해결하는 데 뛰어납니다.", "성향"="고충이나 문제가 발생해도 위축되지 않음", "행동 양상"="고충을 유발한 원인이나 장애를 일으키는 시스템 버그를 찾아 무엇이 문제인지 진단함", "기여하는 것"="문제 있는 상황에 대한 용기와 창의성", "필요로 하는 것(요구 사항)"="반드시 해결해야 하는 문제", "좋아하는 것(가치)"="해결책 찾기", "싫어하는 것(가치)"="무시하면 문제가 사라질 것이라는 생각", "은유/이미지"="탐정, 문제점 조사와 해결책 찾기", "장벽(Barrier Label)"="모든 상황에서 문제점을 찾는 경향이 있기 때문에 다른 사람에게 부정적으로 비추어짐", "adj"="문제에 주의를 기울이는\n의욕이 넘치는\n조사에 능한\n약점에 주의를 기울이는\n즉각 반응하는\n겁이 없는\n통찰력이 있는", "noun"="해결사\n진단자\n문제 해결자\n조사자\n회복시키는 사람\n소생시키는 사람"}]
  out "content comp arr":refnum<vi>[](array[refnum])
  out "contents comp 16":T4
  out "contents comp 15":T4
  out "contents comp 14":T4
  out "contents comp 13":T4
  out "contents comp 12":T4
  out "contents comp 11":T4
  out "contents comp 10":T4
  out "contents comp 9":T4
  out "contents comp 8":T4
  out "contents comp 7":T4
  out "contents comp 6":T4
  out "contents comp 5":T4
  out "contents comp 4":T4
  out "contents comp 3":T4
  out "contents comp 2":T4
  out "가장 길이가 긴 설명.\n화합":string=" 경쟁 우위를 차지하려면 현실적인 관점에서 효율적으로 협업하는 접근 방식이 가장 좋습니다."
  out "contents comp 1":T4
  out "Classify text comp":T4
  out "Classify color comp":u32(colorbox)
  out "Talent comp":T4
  out "테마 대조 재능 index":i32[][](array[numeric])=[[1, 3], [1, 25], [2, 25], [2, 33], [3, 5], [3, 16], [4, 17], [4, 34], [5, 6], [5, 3], [6, 12], [6, 18], [7, 20], [7, 23], [8, 32], [8, 2], [9, 28], [9, 10], [10, 31], [10, 34], [11, 4], [11, 21], [12, 9], [12, 33], [13, 10], [13, 30], [14, 25], [14, 28], [15, 27], [15, 18], [16, 3], [16, 9], [17, 2], [17, 14], [18, 25], [18, 7], [19, 3], [19, 32], [20, 4], [20, 32], [21, 24], [21, 25], [22, 6], [22, 15], [23, 33], [23, 32], [24, 15], [24, 1], [25, 24], [25, 27], [26, 28], [26, 5], [27, 7], [27, 16], [28, 29], [28, 8], [29, 1], [29, 3], [30, 20], [30, 4], [31, 23], [31, 3], [32, 20], [32, 33], [33, 12], [33, 31], [34, 1], [34, 19]]
  out "테마대조 출현 횟수":string[](array[string])=["8_분석", "7_집중", "6_심사숙고", "6_사교성", "5_전략", "5_지적사고", "5_행동", "5_화합", "4_배움", "4_공감", "4_개별화", "4_책임", "4_포용", "4_최상화", "4_절친", "4_적응", "4_연결성", "4_정리", "4_존재감", "4_미래지향", "4_체계", "4_승부", "4_복구", "3_자기확신", "3_발상", "3_수집", "3_긍정", "3_회고", "3_신념", "3_성취", "2_커뮤니케이션", "2_개발", "2_공정성", "2_주도력", "0_"]
  out "contents deep title arr":refnum<vi>[](array[refnum])
  out "contents deep arr":refnum<vi>[](array[refnum])
  out "contents deep 3":T4
  out "contents deep 4":T4
  out "contents deep 5":T4
  out "contents deep 6":T4
  out "contents deep 7":T4
  out "contents deep 8":T4
  out "contents deep 2":T4
  out "contents deep 1":T4
  out "contents deep title 2":T4
  out "contents deep title 8":T4
  out "contents deep title 7":T4
  out "contents deep title 6":T4
  out "contents deep title 5":T4
  out "contents deep title 4":T4
  out "contents deep title 3":T4
  out "toggle data":string
  out "img space":i16
  out "subset rect":T5={"left"=0, "top"=0, "right"=380, "bottom"=620}
  out "summary deep":T4
  out "Classify text deep":T4
  out "Classify color deep":u32(colorbox)
  out "Talent deep":T4
  out "contents deep title 1":T4
  out "adj array":refnum<vi>[](array[refnum])
  out "adj 14":T4
  out "adj 13":T4
  out "adj 12":T4
  out "adj 11":T4
  out "adj 10":T4
  out "adj 9":T4
  out "adj 8":T4
  out "adj 7":T4
  out "adj 6":T4
  out "adj 5":T4
  out "adj 4":T4
  out "adj 3":T4
  out "adj 2":T4
  out "Classify text":T4
  out "Classify color":u32(colorbox)
  out "adj 1":T4
  out "Talent":T4
  out "Background":u32(colorbox)=16777226
  out "Background black":u32(colorbox)
  out "Background deep":u32(colorbox)=16777225
  out "Background black deep":u32(colorbox)
  out "Background comp":u32(colorbox)=16777225
  out "Background black comp":u32(colorbox)
  # "형용사"
  # "테마 조합"
  # "테마 대조"
  # "나를 가장 잘 드러내는 말"
  # "+"
  # "테마 설명 분석"
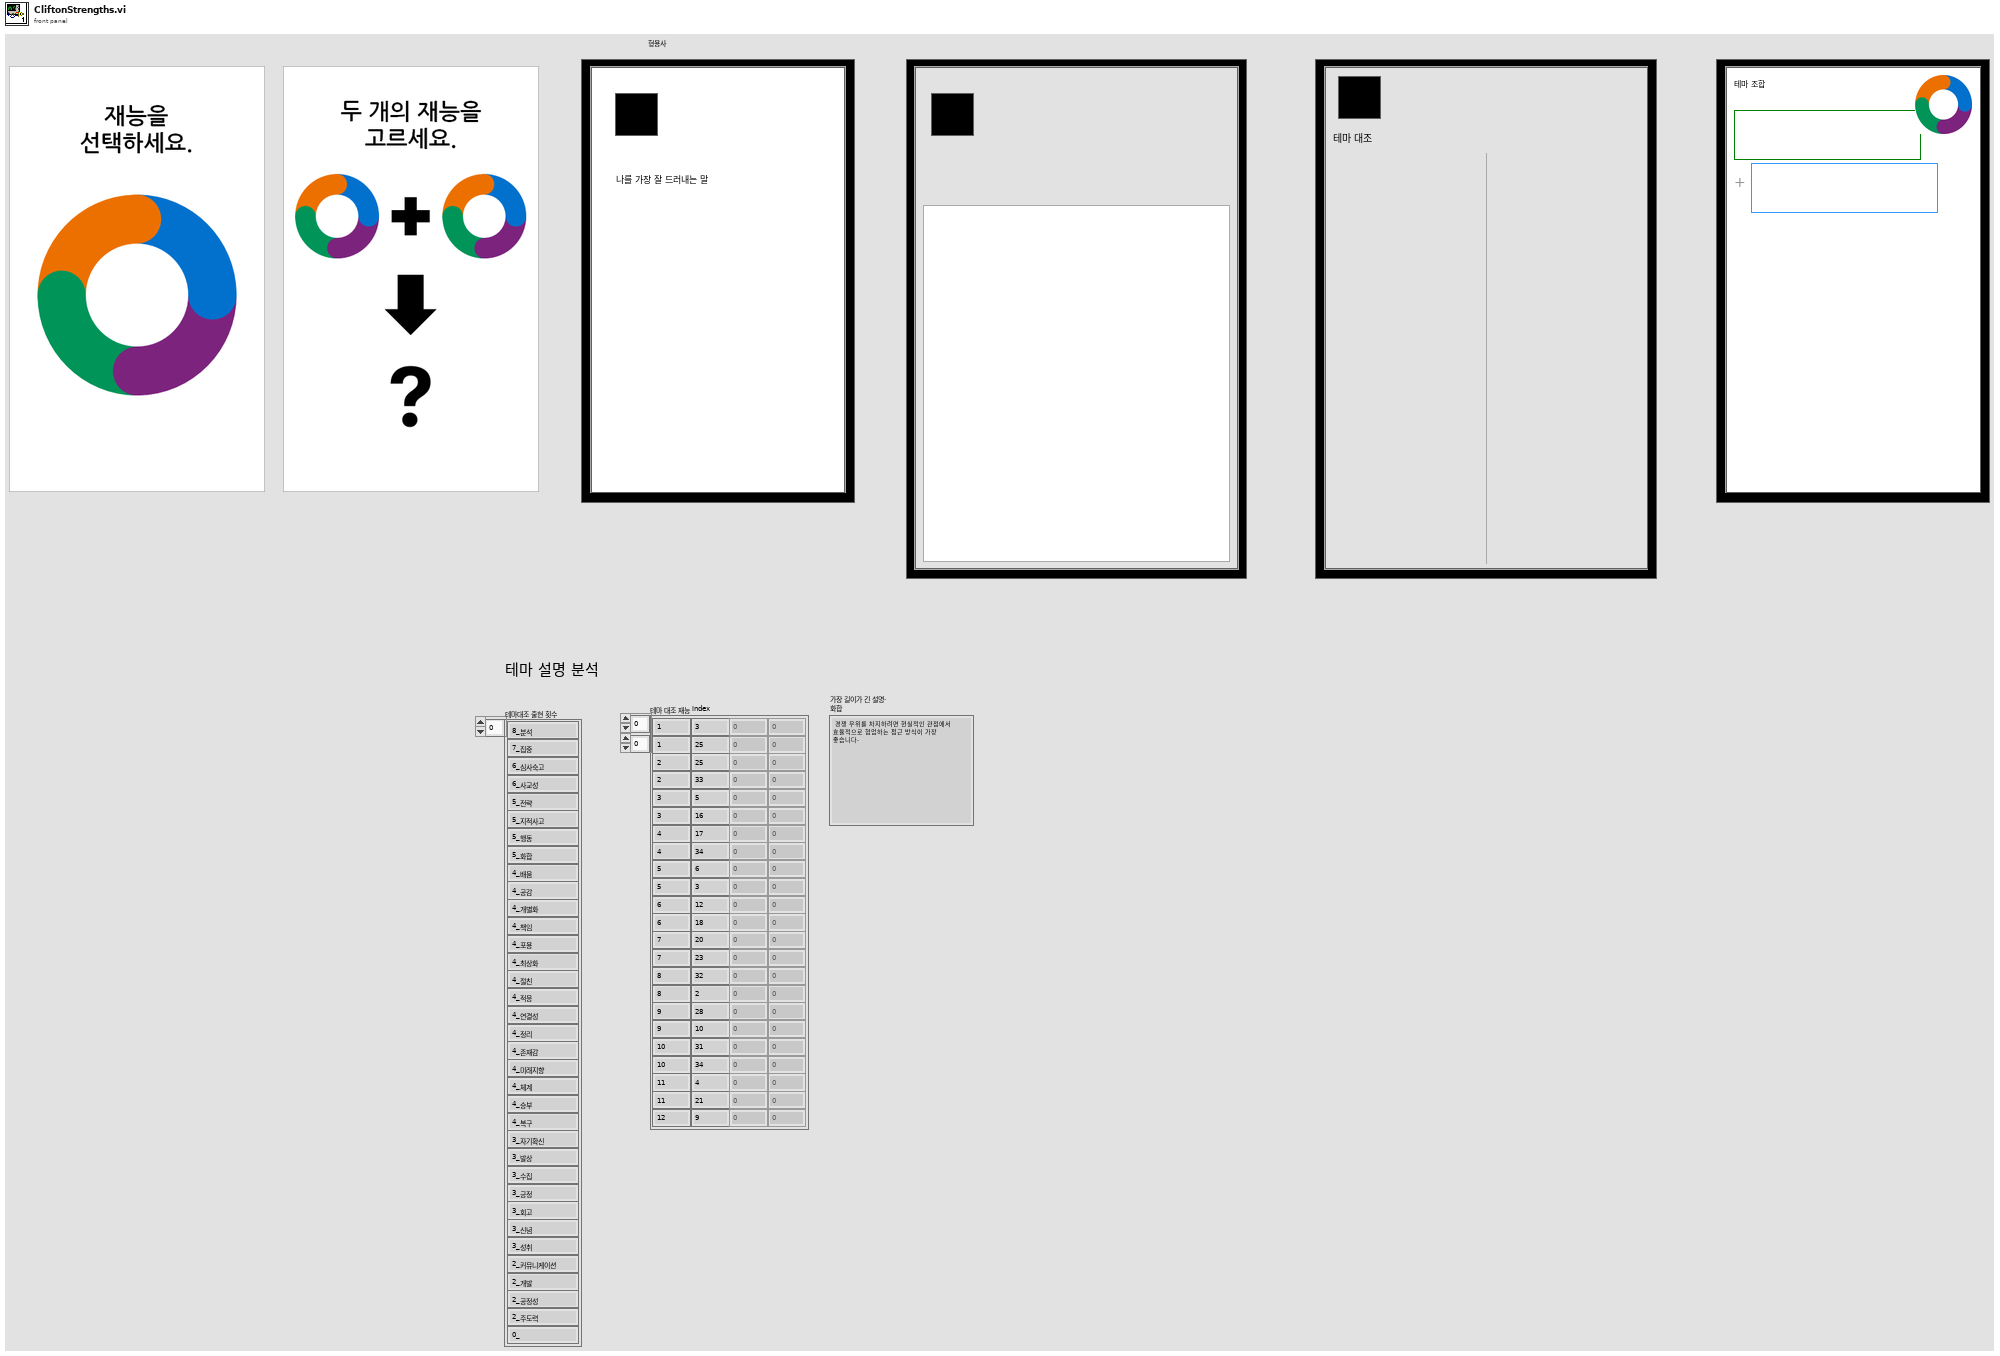
[diagram p1: front panel]
types:
  T1 = typedef "ctrl_CB_talent.ctl" = string
  T2 = typedef "ctrl_CB_description.ctl" = string
  T3 = cluster{"Talent":string, "Talent_eng":string, "Classify text":string, "설명":string, "성향":string, "행동 양상":string, "기여하는 것":string, "필요로 하는 것(요구 사항)":string, "좋아하는 것(가치)":string, "싫어하는 것(가치)":string, "은유/이미지":string, "장벽(Barrier Label)":string, "adj":string, "noun":string}[]
  T4 = typedef "ctrl_white_stringBox.ctl" = string
  T5 = cluster{"left":i16, "top":i16, "right":i16, "bottom":i16}
  T6 = typedef "ctrl_enum_overview.ctl" = enum16{"data1", "data2", "preset1", "preset2", "preset3", "preset4", "make card"}
  T7 = typedef "ctrl_enum_adj.ctl" = enum16{"(interact)img pos size", "(interact)edit title", "(interact)edit contents", "(interact)capture img", "(deep)img pos size", "(deep)edit title", "(deep)edit contents", "(deep)capture img", "(comp)img pos size", "(comp)edit title", "(comp)edit contents", "(comp)capture img", "(CB)img pos size", "(CB)edit title", "(CB)edit contents", "(CB)capture img"}
  T8 = typedef "LVPointTypeDef.ctl" = cluster{"Horizontal":i16, "Vertical":i16}
  T9 = typedef "LVBoundsTypeDef.ctl" = cluster{"Width":u32, "Height":u32}
  T10 = typedef "imagedata.ctl" = cluster{"image type":i32, "image depth":i32, "image":u8[], "mask":u8[], "colors":u32[], "Rectangle":cluster{"left":i16, "top":i16, "right":i16, "bottom":i16}}
  T11 = cluster{"Talent":string, "Talent_eng":string, "Classify text":string, "설명":string, "성향":string, "행동 양상":string, "기여하는 것":string, "필요로 하는 것(요구 사항)":string, "좋아하는 것(가치)":string, "싫어하는 것(가치)":string, "은유/이미지":string, "장벽(Barrier Label)":string, "adj":string, "noun":string}
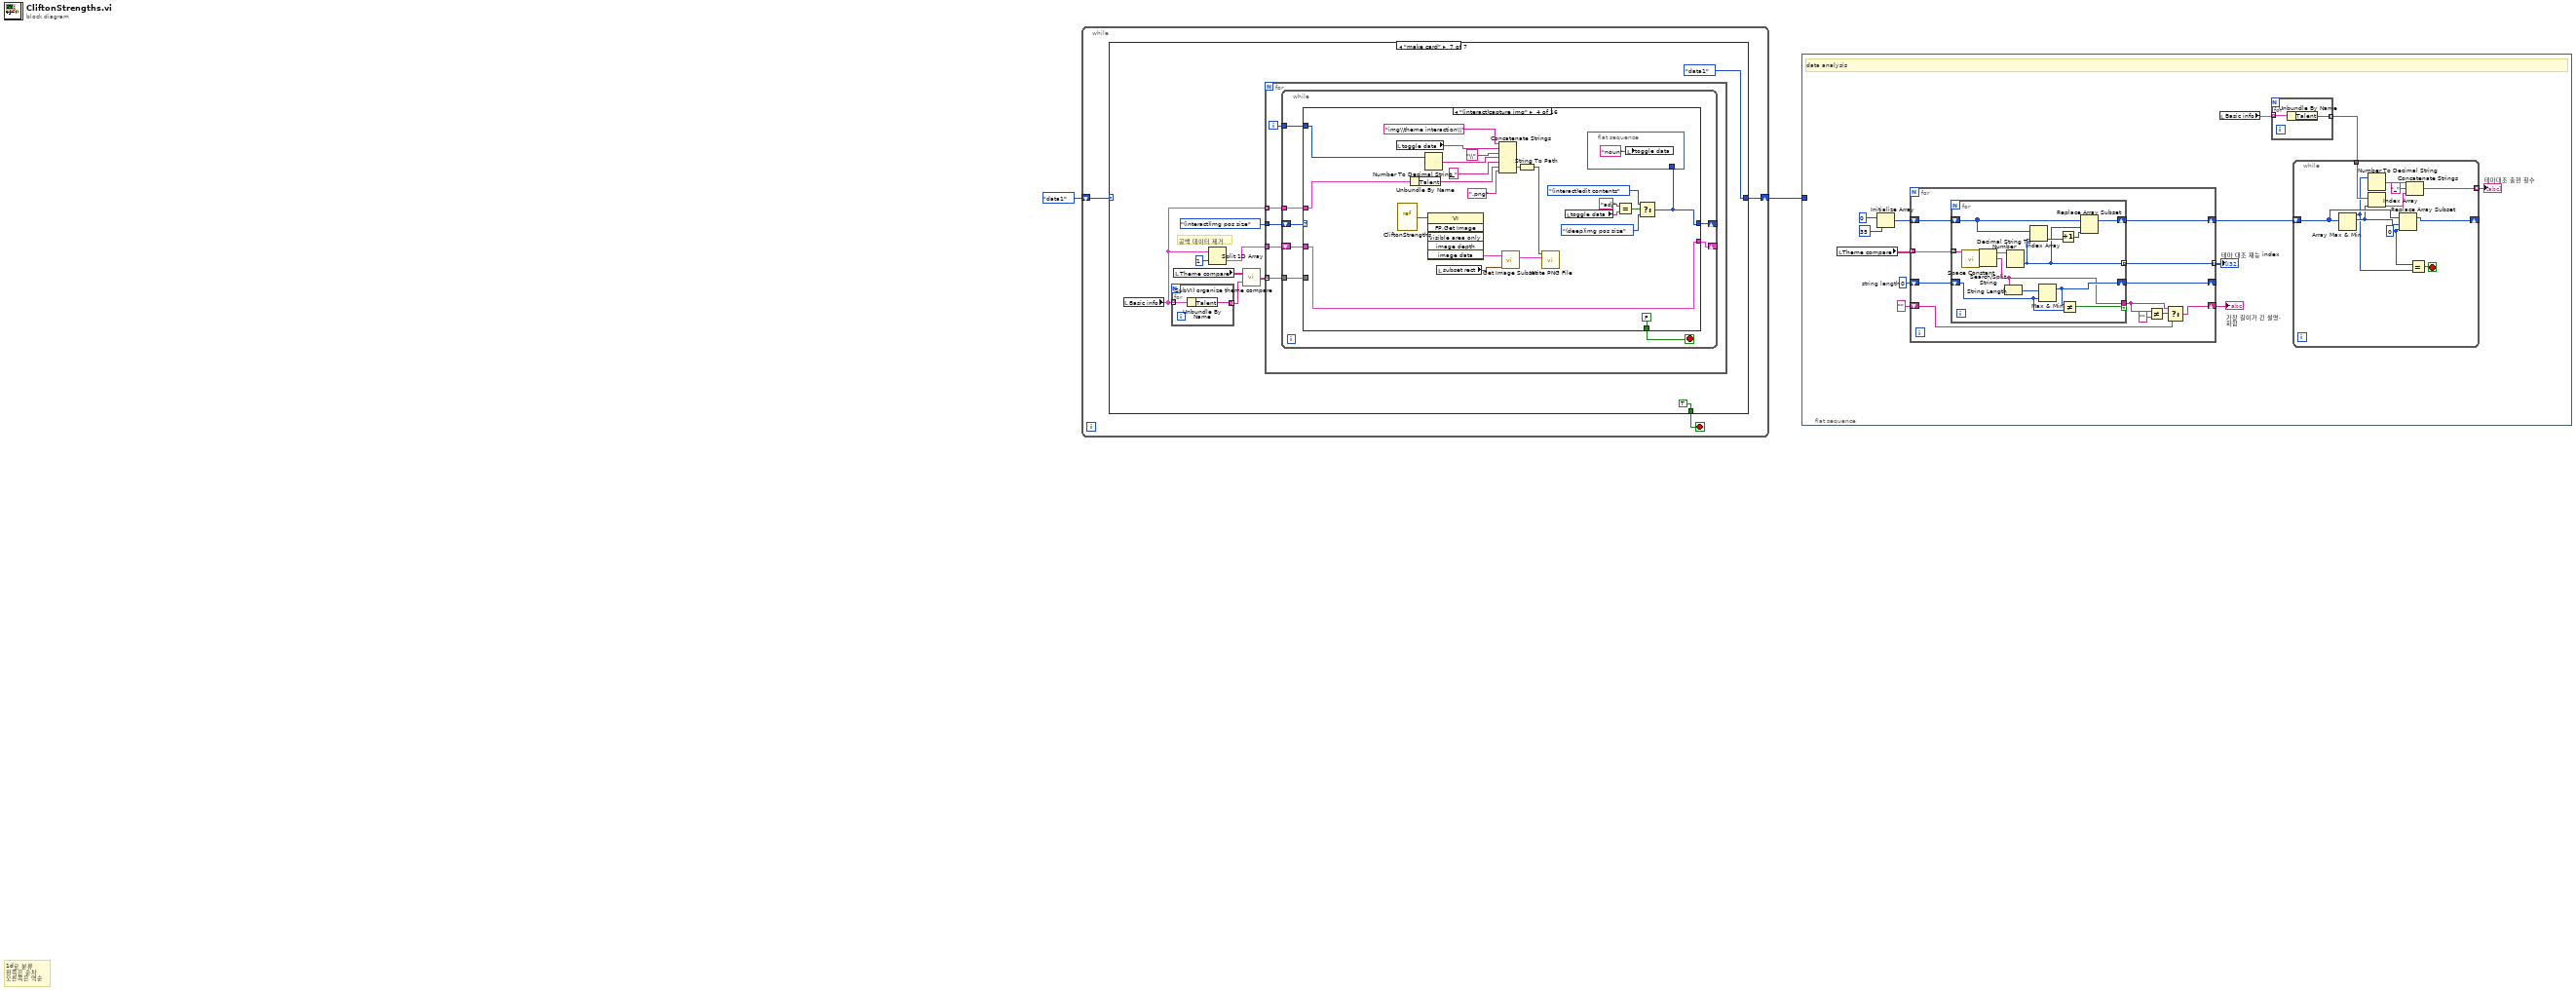
[diagram p0: block diagram]
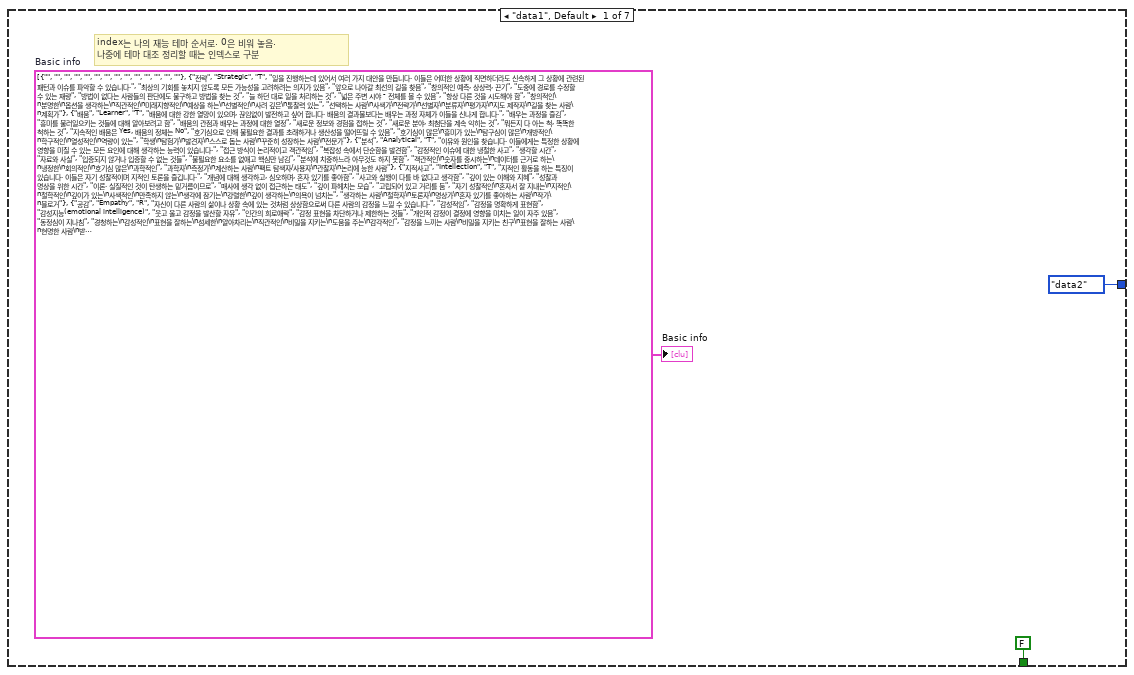
[diagram p2: hidden frame]
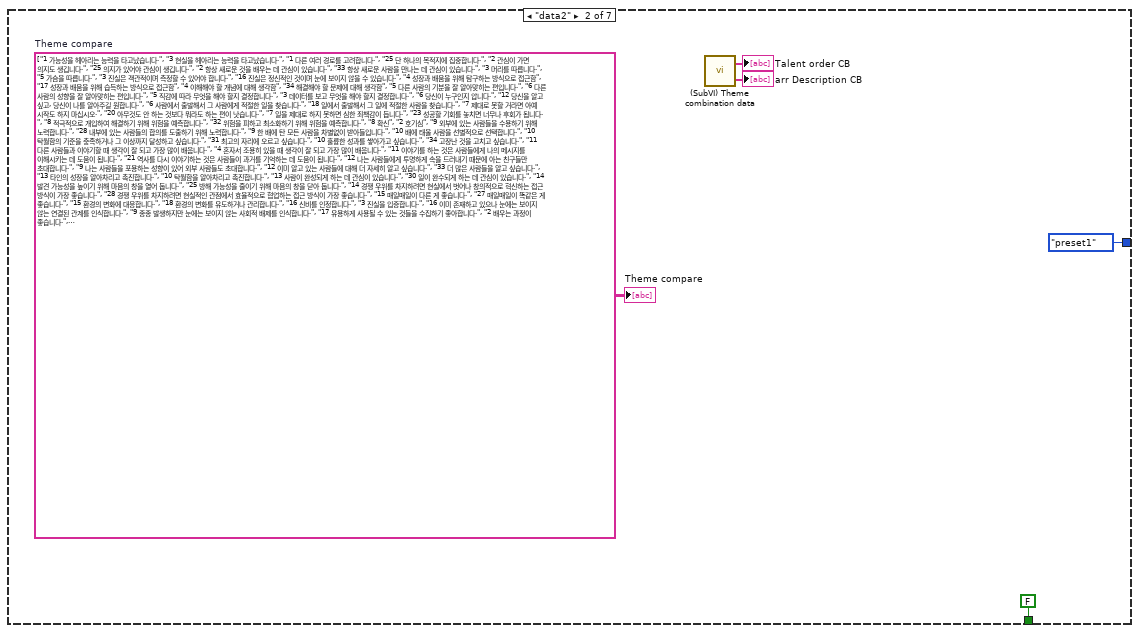
[diagram p3: hidden frame]
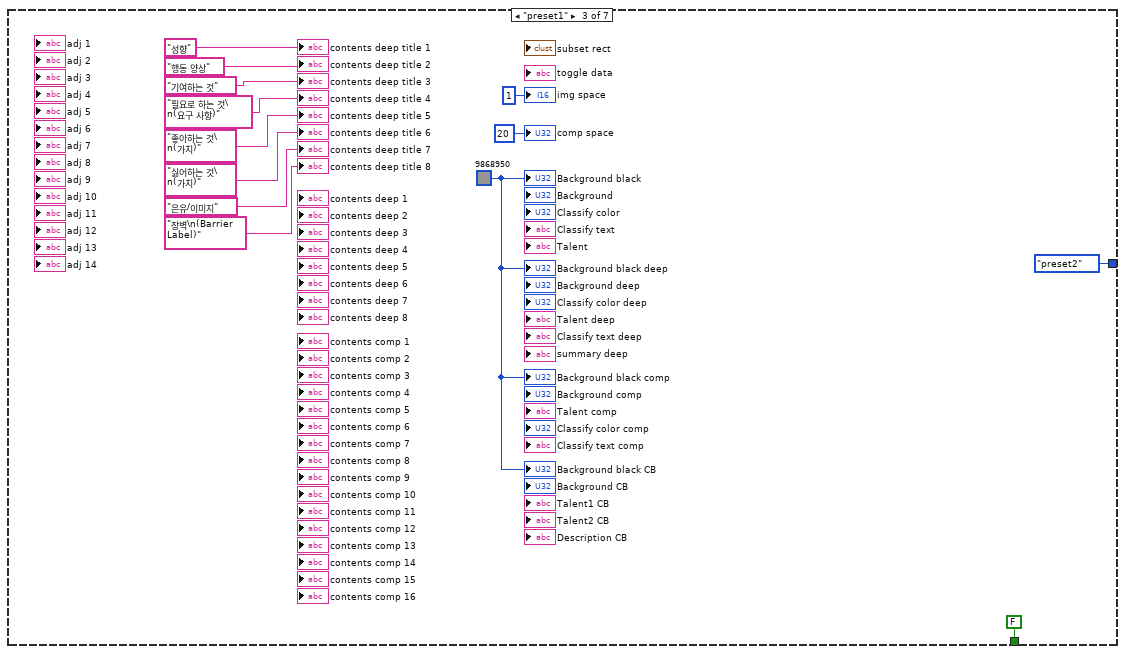
[diagram p4: hidden frame]
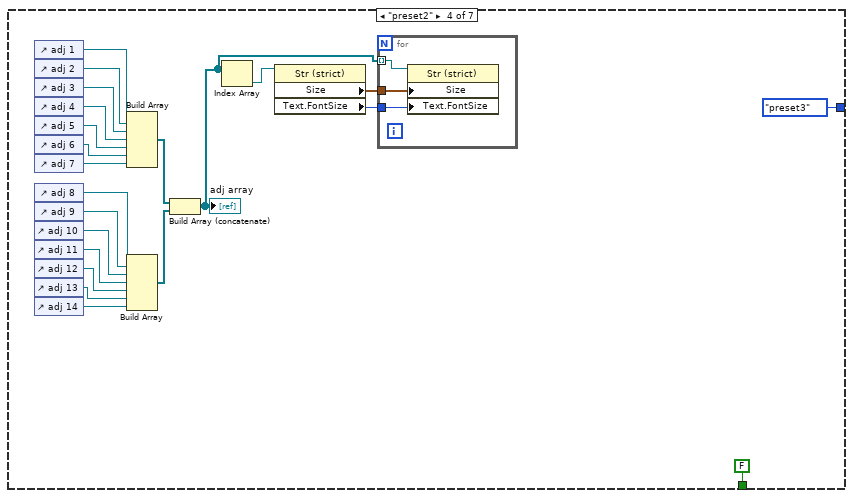
[diagram p5: hidden frame]
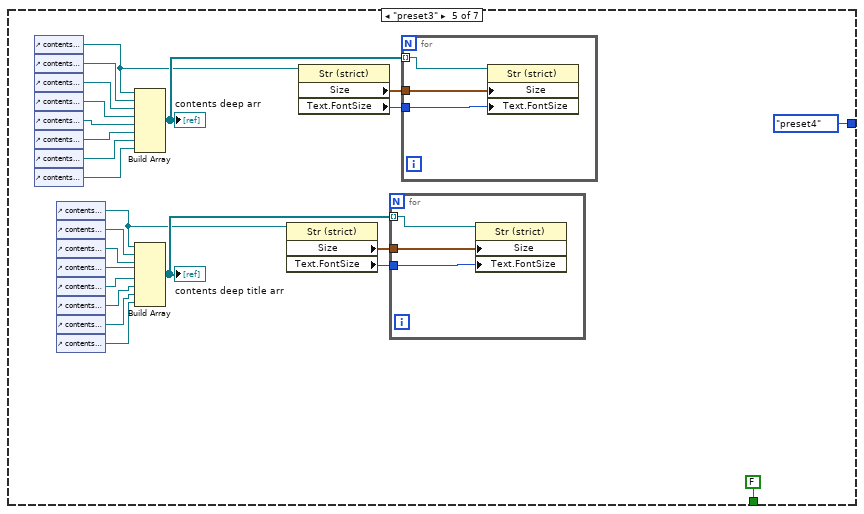
[diagram p6: hidden frame]
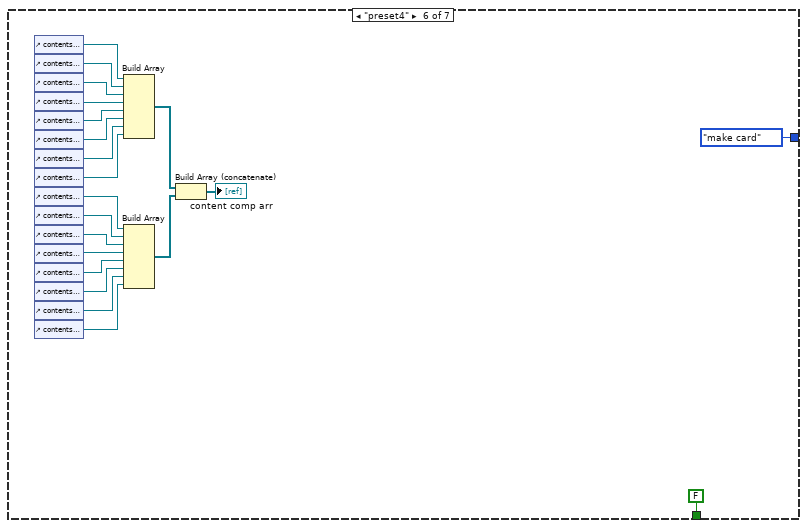
[diagram p7: hidden frame]
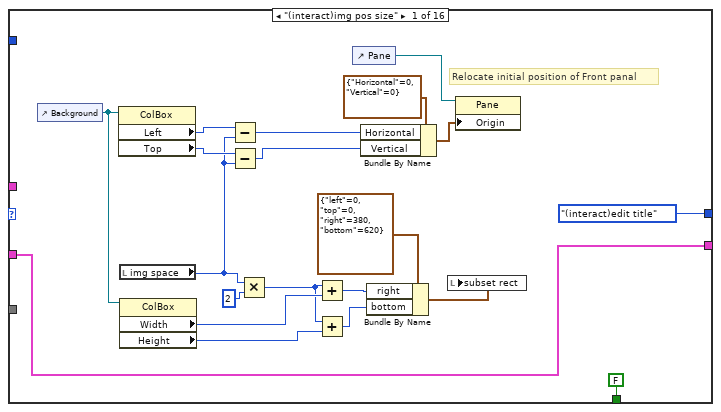
[diagram p8: hidden frame]
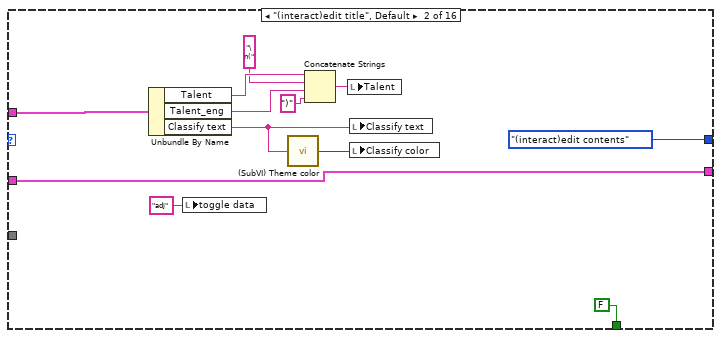
[diagram p9: hidden frame]
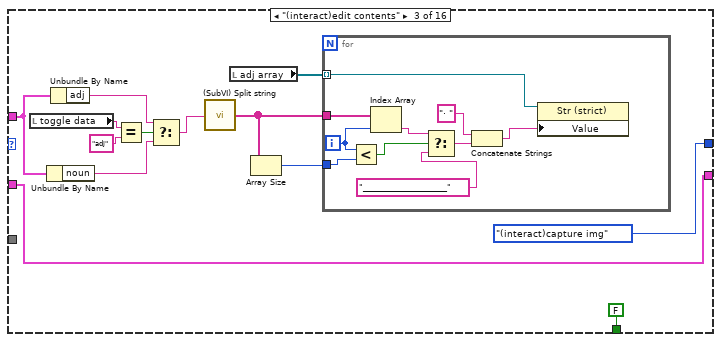
[diagram p10: hidden frame]
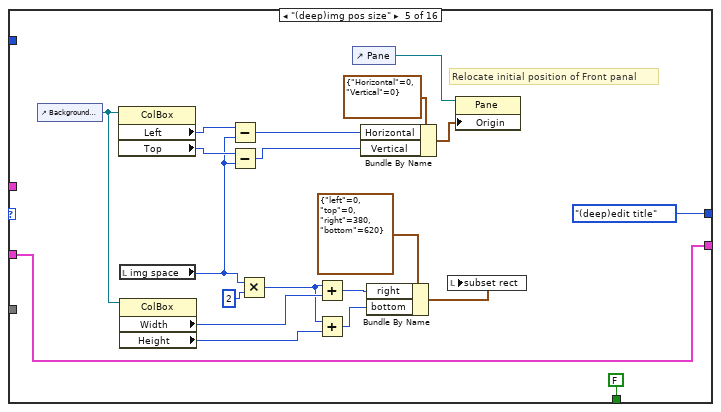
[diagram p11: hidden frame]
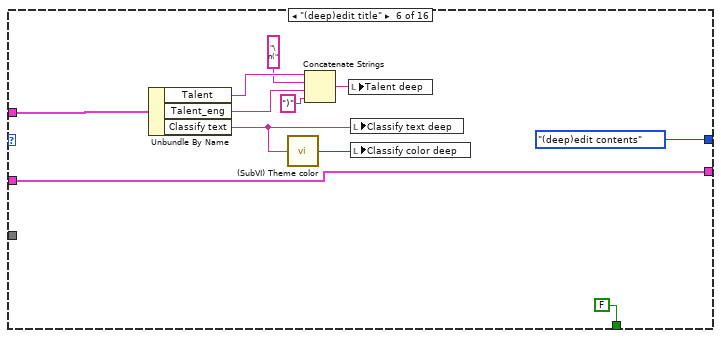
[diagram p12: hidden frame]
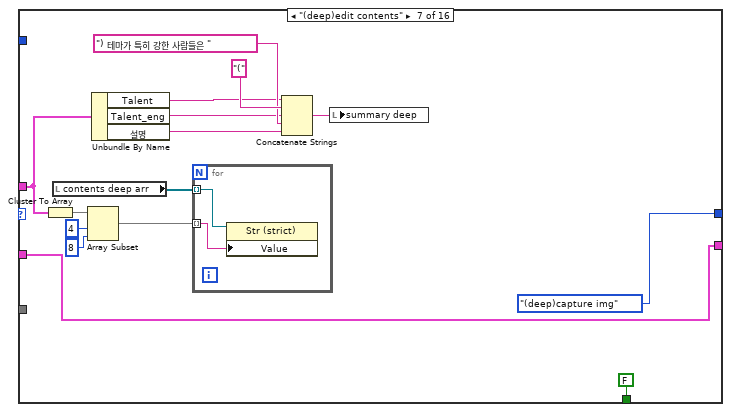
[diagram p13: hidden frame]
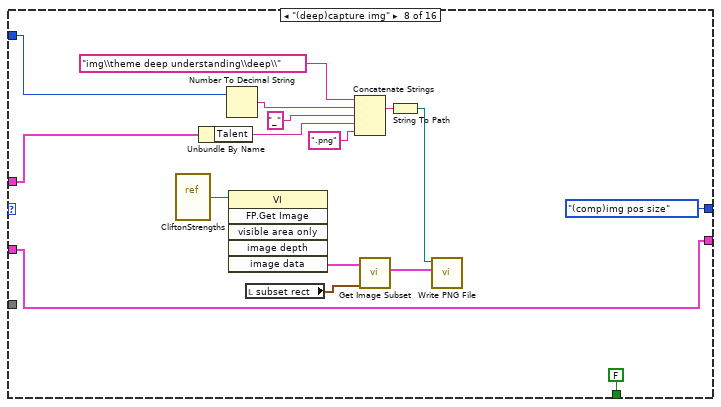
[diagram p14: hidden frame]
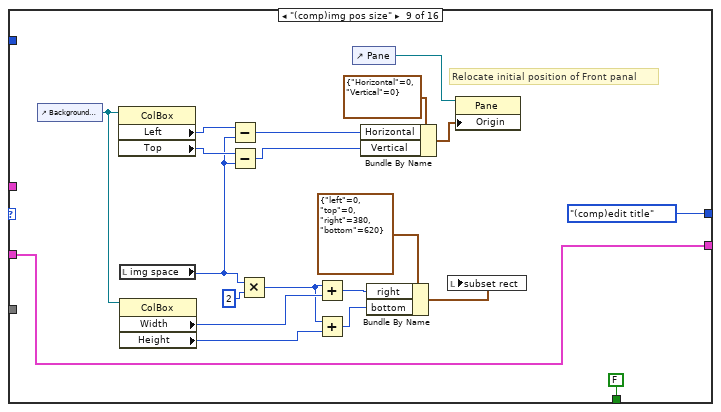
[diagram p15: hidden frame]
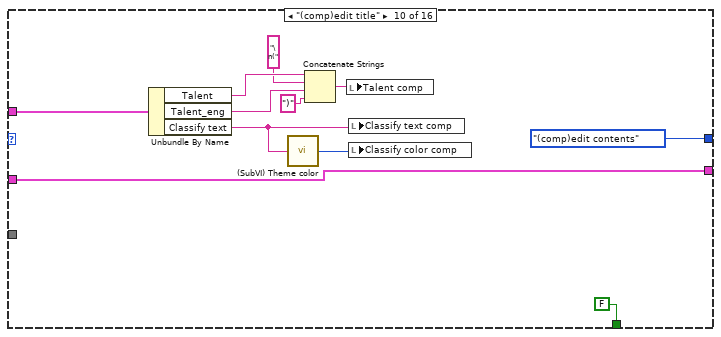
[diagram p16: hidden frame]
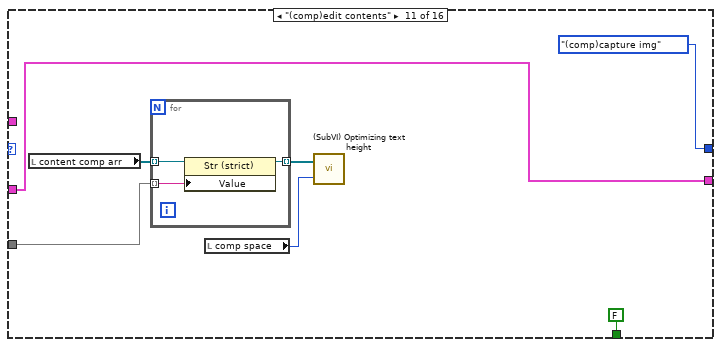
[diagram p17: hidden frame]
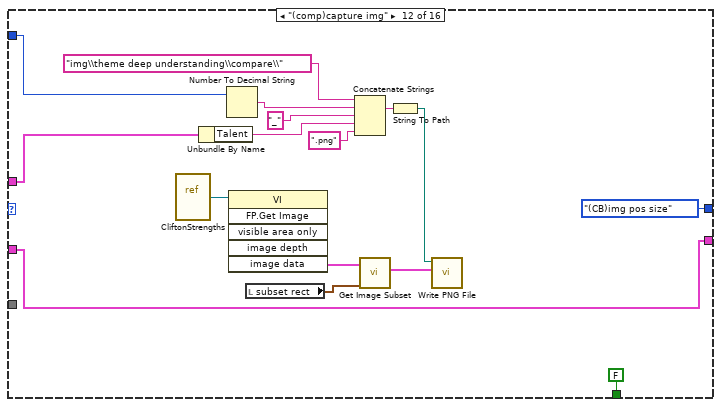
[diagram p18: hidden frame]
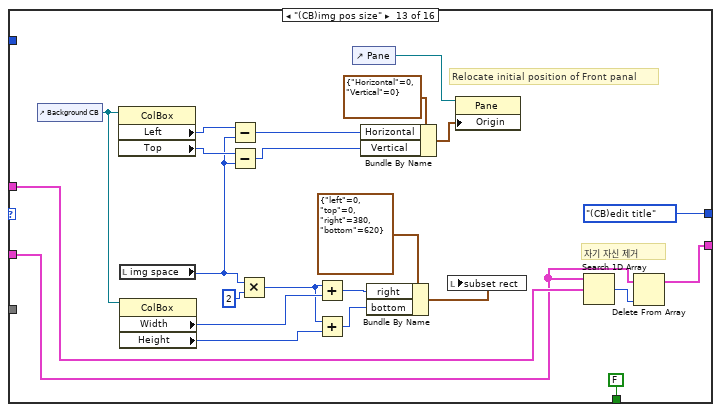
[diagram p19: hidden frame]
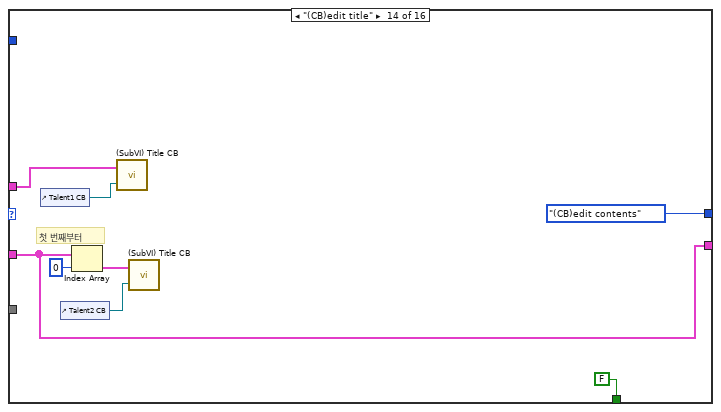
[diagram p20: hidden frame]
diagram:
  # "1d로 분류\n왼쪽은 순차\n오른쪽은 역순"
  n1 = while {
    shift-right: [w3] -> w1
    shift-left: ctrl_enum_overview."data1" ("Enum") -> [w5]
    stop <- w4 stop-if-true
    n2 = case shown="\"make card\"" w5 {
      tunnel: [FALSE FALSE FALSE FALSE FALSE FALSE TRUE] -> w4
      tunnel: [ctrl_enum_overview."data2" ("Enum") ctrl_enum_overview."preset1" ("Enum") ctrl_enum_overview."preset2" ("Enum") ctrl_enum_overview."preset3" ("Enum") ctrl_enum_overview."preset4" ("Enum") ctrl_enum_overview."make card" ("Enum") ctrl_enum_overview."data1" ("Enum")] -> w3
      frame "data1", Default {
        w8 = T3 [{"Talent"="", "Talent_eng"="", "Classify text"="", "설명"="", "성향"="", "행동 양상"="", "기여하는 것"="", "필요로 하는 것(요구 사항)"="", "좋아하는 것(가치)"="", "싫어하는 것(가치)"="", "은유/이미지"="", "장벽(Barrier Label)"="", "adj"="", "noun"=""}, {"Talent"="전략", "Talent_eng"="Strategic", "Classify text"="T", "설명"="일을 진행하는데 있어서 여러 가지 대안을 만듭니다. 이들은 어떠한 상황에 직면하더라도 신속하게 그 상황에 관련된 패턴과 이슈를 파악할 수 있습니다.", "성향"="최상의 기회를 놓치지 않도록 모든 가능성을 고려하려는 의지가 있음", "행동 양상"="앞으로 나아갈 최선의 길을 찾음", "기여하는 것"="창의적인 예측, 상상력, 끈기", "필요로 하는 것(요구 사항)"="도중에 경로를 수정할 수 있는 재량", "좋아하는 것(가치)"="방법이 없다는 사람들의 판단에도 불구하고 방법을 찾는 것", "싫어하는 것(가치)"="늘 하던 대로 일을 처리하는 것", "은유/이미지"="넓은 주변 시야 - 전체를 볼 수 있음", "장벽(Barrier Label)"="항상 다른 것을 시도해야 함", "adj"="창의적인\n분명한\n옵션을 생각하는\n직관적인\n미래지향적인\n예상을 하는\n선별적인\n사려 깊은\n통찰력 있는", "noun"="선택하는 사람\n사색가\n전략가\n선별자\n분류자\n평가자\n지도 제작자\n길을 찾는 사람\n계획가"}, {"Talent"="배움", "Talent_eng"="Learner", "Classify text"="T", "설명"="배움에 대한 강한 열망이 있으며, 끊임없이 발전하고 싶어 합니다. 배움의 결과물보다는 배우는 과정 자체가 이들을 신나게 합니다.", "성향"="배우는 과정을 즐김", "행동 양상"="흥미를 불러일으키는 것들에 대해 알아보려고 함", "기여하는 것"="배움의 관점과 배우는 과정에 대한 열정", "필요로 하는 것(요구 사항)"="새로운 정보와 경험을 접하는 것", "좋아하는 것(가치)"="새로운 분야, 최첨단을 계속 익히는 것", "싫어하는 것(가치)"="뭐든지 다 아는 척, 똑똑한 척하는 것", "은유/이미지"="지속적인 배움은 Yes, 배움의 정체는 No", "장벽(Barrier Label)"="호기심으로 인해 불필요한 결과를 초래하거나 생산성을 떨어뜨릴 수 있음", "adj"="호기심이 많은\n흥미가 있는\n탐구심이 많은\n개방적인\n학구적인\n열성적인\n역량이 있는", "noun"="학생\n탐험가\n발견자\n스스로 돕는 사람\n꾸준히 성장하는 사람\n전문가"}, {"Talent"="분석", "Talent_eng"="Analytical", "Classify text"="T", "설명"="이유와 원인을 찾습니다. 이들에게는 특정한 상황에 영향을 미칠 수 있는 모든 요인에 대해 생각하는 능력이 있습니다.", "성향"="접근 방식이 논리적이고 객관적임", "행동 양상"="복잡성 속에서 단순함을 발견함", "기여하는 것"="감정적인 이슈에 대한 냉철한 사고", "필요로 하는 것(요구 사항)"="생각할 시간", "좋아하는 것(가치)"="자료와 사실", "싫어하는 것(가치)"="입증되지 않거나 입증할 수 없는 것들", "은유/이미지"="불필요한 요소를 없애고 핵심만 남김", "장벽(Barrier Label)"="분석에 치중하느라 아무것도 하지 못함", "adj"="객관적인\n숫자를 중시하는\n데이터를 근거로 하는\n냉정한\n회의적인\n호기심 많은\n과학적인", "noun"="과학자\n측정가\n계산하는 사람\n팩트 탐색자/사용자\n관찰자\n논리에 능한 사람"}, {"Talent"="지적사고", "Talent_eng"="Intellection", "Classify text"="T", "설명"="지적인 활동을 하는 특징이 있습니다. 이들은 자기 성찰적이며 지적인 토론을 즐깁니다.", "성향"="개념에 대해 생각하고, 심오하며, 혼자 있기를 좋아함", "행동 양상"="사고와 실행이 다를 바 없다고 생각함", "기여하는 것"="깊이 있는 이해와 지혜", "필요로 하는 것(요구 사항)"="성찰과 명상을 위한 시간", "좋아하는 것(가치)"="이론. 실질적인 것이 탄생하는 밑거름이므로", "싫어하는 것(가치)"="매사에 생각 없이 접근하는 태도", "은유/이미지"="깊이 파헤치는 모습", "장벽(Barrier Label)"="고립되어 있고 거리를 둠", "adj"="자기 성찰적인\n혼자서 잘 지내는\n지적인\n철학적인\n깊이가 있는\n사색적인\n만족하지 않는\n생각에 잠기는\n강렬한\n깊이 생각하는\n의욕이 넘치는", "noun"="생각하는 사람\n철학자\n토론자\n명상가\n혼자 있기를 좋아하는 사람\n작가\n블로거"}, {"Talent"="공감", "Talent_eng"="Empathy", "Classify text"="R", "설명"="자신이 다른 사람의 삶이나 상황 속에 있는 것처럼 상상함으로써 다른 사람의 감정을 느낄 수 있습니다.", "성향"="감성적임", "행동 양상"="감정을 명확하게 표현함", "기여하는 것"="감성지능(emotional intelligence)", "필요로 하는 것(요구 사항)"="웃고 울고 감정을 발산할 자유", "좋아하는 것(가치)"="인간의 희로애락", "싫어하는 것(가치)"="감정 표현을 차단하거나 제한하는 것들", "은유/이미지"="개인적 감정이 결정에 영향을 미치는 일이 자주 있음", "장벽(Barrier Label)"="동정심이 지나침", "adj"="경청하는\n감성적인\n표현을 잘하는\n섬세한\n알아차리는\n직관적인\n비밀을 지키는\n도움을 주는\n감각적인", "noun"="감정을 느끼는 사람\n비밀을 지키는 친구\n표현을 잘하는 사람\n현명한 사람\n받아들이는 사람\n경청하는 사람\n공감하는 사람"}, {"Talent"="개별화", "Talent_eng"="Individualization", "Classify text"="R", "설명"="각 사람이 지닌 독특한 개성에 흥미를 느낍니다. 이들은 서로 다른 사람들이 어떻게 협력하여 생산적으로 일할 수 있는지 파악하는 데 재능이 있습니다.", "성향"="상황을 각 개인에 맞춰줌", "행동 양상"="인간의 다양성이 지닌 문제점보다는 잠재력에 주목함", "기여하는 것"="사람을 잘 이해하여 인력 배치에 도움을 줌", "필요로 하는 것(요구 사항)"="개인 맞춤형 기대치 설정", "좋아하는 것(가치)"="사람들이 각자 가장 잘하는 일을 하게 되는 것", "싫어하는 것(가치)"="한 가지 방식을 모든 상황에 적용하는 접근 방식", "은유/이미지"="배역 담당자 - 배우들에 대해 알고 있는 사항을 활용함", "장벽(Barrier Label)"="개인의 요구를 충족하기 위해 집단의 요구를 희생함", "adj"="알아차리는\n독특한\n직관력이 있는\n사람을 중시하는\n강점을 중시하는\n기민한\n공정한\n정확한\n통찰력이 있는\n다양성을 중시하는", "noun"="개인화하는 사람\n관찰자\n받아들이는 사람\n알아차리는 사람\n물색하는 사람\n인류학자\n소설가\n전기 작가"}, {"Talent"="책임", "Talent_eng"="Responsibility", "Classify text"="E", "설명"="자신이 하겠다고 약속한 것들에 대해서 강한 주인의식(ownership)을 느낍니다. 이들은 정직성과 충실함 같은 가치관을 매우 중요시 합니다.", "성향"="일을 완수하리라 믿고 맡길 수 있는 사람임", "행동 양상"="약속을 최선을 다해 끝까지 지킴", "기여하는 것"="신뢰와 충실함", "필요로 하는 것(요구 사항)"="주인 의식을 가질 수 있는 재량", "좋아하는 것(가치)"="다른 사람들의 존경", "싫어하는 것(가치)"="사람들을 실망시키고 사람들에게 실망하는 것", "은유/이미지"="무관심한 세입자가 아닌 진지한 소유주", "장벽(Barrier Label)"="거절하지 못하고, 쉽게 놓지 못함", "adj"="근면한\n양심적인\n판단을 하는\n충성스러운\n의욕적인\n임무를 완수하는\n믿음직스러운\n진지한\n헌신적인\n자기 희생적인\n즉각 반응하는\n독립적인", "noun"="주인의식이 있는 사람\n노력하는 사람\n섬김의 정신이 강한 사람\n응답하는 사람\n완벽주의자\n심판\n자원자\n제어하는 사람"}, {"Talent"="자기확신", "Talent_eng"="Self-Assurance", "Classify text"="I", "설명"="위험을 감수하고 삶을 이끌어가는 자신의 능력에 대한 자신감을 가지고 있습니다. 이들에게는 자신의 의사결정에 확신을 갖게 하는 내면의 나침반이 있습니다.", "성향"="외부적으로 불확실한 상황에서도 자신감을 유지함", "행동 양상"="영향을 받기보다 영향력을 행사하고자 함", "기여하는 것"="필요한 위험을 감수할 의지", "필요로 하는 것(요구 사항)"="일방적, 독립적으로 활동할 수 있는 재량", "좋아하는 것(가치)"="운명은 스스로 결정하는 것이라는 태도", "싫어하는 것(가치)"="다른 사람의 지시", "은유/이미지"="마음의 나침반, 내면의 북소리에 맞춰 행진하는 모습", "장벽(Barrier Label)"="오만, 지나친 자신감, 자기 만족", "adj"="독립적인\n확신하는\n자신감 있는\n자의식 있는\n자립적인\n본능적인\n강렬한\n통제하는\n안정적인\n집요한", "noun"="인플루엔서\n통제자\n감독\n위험 감수자\n리더"}, {"Talent"="포용", "Talent_eng"="Includer", "Classify text"="R", "설명"="다른 사람을 받아들입니다. 이들은 소외되었다고 느끼는 사람을 알아차리고 그들을 포용하기 위해 노력합니다.", "성향"="배제된 사람을 알아차리고 그로 인해 초래될 영향을 이해함", "행동 양상"="가진 자와 못 가진 자의 격차를 줄임", "기여하는 것"="다양성 수용에 대한 높은 수준의 관용", "필요로 하는 것(요구 사항)"="누구나 받아들일 수 있는 여지", "좋아하는 것(가치)"="동화와 통합", "싫어하는 것(가치)"="패거리 문화", "은유/이미지"="모토 - 여기서는 누구나 환영합니다", "장벽(Barrier Label)"="무분별함", "adj"="기꺼이 받아들이는\n인내심이 있는\n상호적인\n직관력이 있는\n타인 지향적인\n반갑게 맞이하는\n세심한\n통합하는", "noun"="수용가\n용인하는 사람\n초청자\n환영하는 사람\n동화시키는 사람\n장벽을 허무는 사람"}, {"Talent"="최상화", "Talent_eng"="Maximizer", "Classify text"="I", "설명"="개인이나 집단의 탁월성을 자극하기 위해 그들의 강점에 초점을 맞춥니다. 이들은 좋은 것을 최상의 것으로 전환시킬 방법을 찾습니다.", "성향"="탁월성을 이끌어내는 데 전념함", "행동 양상"="강점에 집중하면서 약점을 관리함", "기여하는 것"="품질 지향", "필요로 하는 것(요구 사항)"="양만큼 질도 중시되어야 함", "좋아하는 것(가치)"="최대의 ROI(Return on Investment, 투자 대비 수익)", "싫어하는 것(가치)"="약점을 고치려는 집착", "은유/이미지"="'좋음'에서 '탁월함'으로, Good-Better-Best", "장벽(Barrier Label)"="까다롭고 만족을 모름", "adj"="선별적인\n강점을 중시하는\n품질을 중시하는\n결과를 중시하는\n강점에 매료되는\n탁월함을 의식하는\n까다로운\n판단을 하는\n가려내는\n만족하지 않는", "noun"="리더\n추진가\n명확하게 밝히는 사람\n설득자\n파이터\n도전자\n요구가 많은 사람\n완벽주의자\n품질 관리자"}, {"Talent"="커뮤니케이션", "Talent_eng"="Communication", "Classify text"="I", "설명"="대체로 쉽게 자신의 생각을 말로 표현합니다. 이들은 대화와 발표에 능합니다.", "성향"="말솜씨가 있음", "행동 양상"="말을 통해 타인과 관계를 구축함", "기여하는 것"="사람들이 들어야 할 메시지에 주의를 집중시킴", "필요로 하는 것(요구 사항)"="반응해주는 사람들, 청중", "좋아하는 것(가치)"="이야기와 이야기꾼", "싫어하는 것(가치)"="표현하지 못한 경험", "은유/이미지"="침묵은 금이 아님", "장벽(Barrier Label)"="수다스러움", "adj"="말하기 좋아하는\n발표를 잘하는\n언어 능력이 있는\n투명한\n상호적인\n대화에 능한\n표현력이 뛰어난\n사로잡는\n재미있는", "noun"="말하는 사람\n발표자\n대화에 능한 사람\n스토리텔러\n말솜씨가 좋은 사람\n설명하는 사람\n작가"}, {"Talent"="절친", "Talent_eng"="Relator", "Classify text"="R", "설명"="주변 사람들과 깊고 친밀한 관계를 맺는 것을 좋아합니다. 이들은 친밀한 사람들과 함께 목표를 향해 열심히 일하는 데에서 깊은 만족감을 얻습니다.", "성향"="진실되고 믿음직스러움", "행동 양상"="가까운 사람들에 대해 더 많이 알아감", "기여하는 것"="깊이 있고 투명한 대인관계", "필요로 하는 것(요구 사항)"="사람들과 일대일 교류할 수 있는 시간과 기회", "좋아하는 것(가치)"="서로를 챙겨주는 친밀한 상호 관계", "싫어하는 것(가치)"="새로운 사람을 처음 만났을 때의 불편함", "은유/이미지"="서로를 잘 아는 친구", "장벽(Barrier Label)"="파벌에 따른, 정에 이끌린 인사를 함", "adj"="친절한\n배려심 있는\n진정성 있는\n진실된\n친밀한\n투명한\n정직한\n자신을 드러내는", "noun"="친구\n가족\n충직한 사람\n다른 사람을 돌보는 사람"}, {"Talent"="개발", "Talent_eng"="Developer", "Classify text"="R", "설명"="다른 사람의 잠재력을 알아보고 이를 키워줍니다. 이들은 작은 진전의 신호를 알아차리며 사람들이 발전해가는 모습에서 만족을 얻습니다.", "성향"="경험이 부족하고 미숙한 사람들에 대해 인내심이 있음", "행동 양상"="타인의 성장에서 만족감을 느낌", "기여하는 것"="사람의 성장에 헌신할 시간과 에너지", "필요로 하는 것(요구 사항)"="투자할 대상자", "좋아하는 것(가치)"="인간의 잠재력과 진보", "싫어하는 것(가치)"="잠재력이 낭비되거나 실현되지 않는 것", "은유/이미지"="걸음마를 배우는 아기를 인내하며 지켜보는 부모", "장벽(Barrier Label)"="저성과자에게 시간을 낭비함", "adj"="참을성이 있는\n직관력이 있는\n유능한\n격려를 잘하는\n시간과 노력을 투자하는\n타인 지향적인\n관찰력이 있는\n성장을 중시하는\n자기 희생적인\n다른 사람에게 도움을 주는", "noun"="투자자\n코치\n멘토\n교사\n격려하는 사람\n역량을 개발해주는 사람"}, {"Talent"="발상", "Talent_eng"="Ideation", "Classify text"="T", "설명"="아이디어에 매료됩니다. 이들은 보기에는 상관없어 보이는 현상들의 연관성을 찾아낼 수 있습니다.", "성향"="혁신에 내포된 애매모호함과 위험 요소에 영향을 받지 않음", "행동 양상"="고정관념에서 벗어난 사고를 함", "기여하는 것"="새롭고 신선한 시각", "필요로 하는 것(요구 사항)"="통제나 제한없이 가능성을 탐색할 자유", "좋아하는 것(가치)"="완전히 새로운 무엇인가를 제시하는 것", "싫어하는 것(가치)"="늘 하던 일을 하는 것", "은유/이미지"="예술가의 창의력, 비어 있는 캔버스나 백지, 찰흙", "장벽(Barrier Label)"="비현실적임", "adj"="즉흥적인\n창의적인\n혁신적인\n예술적인\n통찰력이 있는\n지략이 풍부한\n활기를 주는", "noun"="발명가\n창조자\n디자이너\n예술가\n혁신자\n브레인스토머\n소설가"}, {"Talent"="적응", "Talent_eng"="Adaptability", "Classify text"="R", "설명"="상황의 흐름에 따라 적응하는 것을 선호합니다. 이들은 일이 생기는 대로 받아들이며 미래에 대해서는 그때 가서 대처하려 하며, '현재'에 충실한 경향이 있습니다.", "성향"="\"지금 바로 여기\"를 중시함", "행동 양상"="당면한 상황에 즉각적으로 대응함", "기여하는 것"="변화가 일어나는 방향으로 기꺼이 따라감", "필요로 하는 것(요구 사항)"="즉각적 대응을 필요로 하는 현재의 압력", "좋아하는 것(가치)"="즉흥성", "싫어하는 것(가치)"="예측 가능성", "은유/이미지"="강물처럼 흐름에 따라감", "장벽(Barrier Label)"="방향성이 없음", "adj"="유연한\n먼저 반응하는\n느긋한\n현재에 집중하는\n순간에 충실한\n즉흥적인\n선뜻 동의하는\n실존주의적인", "noun"="먼저 반응하는 사람\n얼리 어답터\n적응하는 사람\n추종자"}, {"Talent"="연결성", "Talent_eng"="Connectedness", "Classify text"="R", "설명"="모든 것들이 연결되어 있다고 믿습니다. 이들은 우연이란 거의 존재하지 않으며 일어나는 거의 모든 일에는 다 의미가 있다고 믿습니다.", "성향"="인류는 국경과 시간을 초월하는 하나의 가족이라고 생각함", "행동 양상"="부분을 전체로 통합함", "기여하는 것"="생명과 모든 우주 만물의 신비와 경이를 인지하고 감사함", "필요로 하는 것(요구 사항)"="자신보다 더 큰 무언가(가족, 팀, 글로벌 커뮤니티, 우주 등)의 일부가 되는 것", "좋아하는 것(가치)"="삶의 순환, 연결의 끈", "싫어하는 것(가치)"="\"편 가르기\" 사고방식", "은유/이미지"="몸, 마음, 영혼이 연결된 사람", "장벽(Barrier Label)"="괴짜, 뉴에이지 애호가, 현실과 동떨어짐", "adj"="통합하는\n탐구하는\n영적인\n위안을 주는\n직관력이 있는\n신비로운\n철학적인\n상담을 해주는\n경청하는", "noun"="통합가\n다리가 되어 주는 사람\n환경주의자\n인도주의자\n공동체주의자\n통합하는 사람\n사회운동가\n탐구자"}, {"Talent"="수집", "Talent_eng"="Input", "Classify text"="T", "설명"="수집하고 보관하고 싶어합니다. 이들은 정보, 아이디어, 작품이나 심지어 관계도 축적할 수 있습니다.", "성향"="실용적인 자원 수집가", "행동 양상"="다른 사람들에게 유용한 자원이 될 수 있는 것들을 수집함", "기여하는 것"="성장과 성과를 촉진할 수 있는 구체적인 도구", "필요로 하는 것(요구 사항)"="자연스럽게 수집하게 된 자원을 보관할 공간", "좋아하는 것(가치)"="관련성이 높은 실질적인 도움을 제공하는 것", "싫어하는 것(가치)"="다른 사람들에게 유용할 만한 자원을 확보하지 못하는 것", "은유/이미지"="흡수(input)하고 내보내는(output) 스펀지", "장벽(Barrier Label)"="필요도 없는 잡다한 것들을 되는대로 쌓아놓음", "adj"="지략이 풍부한\n수집을 즐기는\n탐구심이 많은\n관대한\n박식한\n정통한\n조사에 능한", "noun"="보관하는 사람\n도서관 사서\n수집가\n흡수하는 사람\n큐레이터\n자원을 수집하는 사람\n전달자"}, {"Talent"="정리", "Talent_eng"="Arranger", "Classify text"="E", "설명"="복잡한 상황을 체계적으로 정리할 수 있는 능력과 함께 이를 보완해주는 유연성도 가지고 있습니다. 이들은 생산성을 최대화하기 위해 모든 구성요소와 자원을 최적으로 정리하는 것을 좋아합니다.", "성향"="변수가 많아도 편안함", "행동 양상"="다른 사람들을 통해 더 효과적이고 효율적으로 업무를 수행함", "기여하는 것"="유연성과 상호작용", "필요로 하는 것(요구 사항)"="역동적인 환경", "좋아하는 것(가치)"="필요한 변화의 시작과 관리", "싫어하는 것(가치)"="필요한 변화에 대한 저항", "은유/이미지"="지휘자, 코디네이터", "장벽(Barrier Label)"="너무 잦은 변경으로 쫓아가기 어려움", "adj"="유연한\n상호적인\n통제를 잘하는\n협력적인\n동시에 여러 가지를 고려하는\n구성에 능한\n즉각적인\n지략이 풍부한", "noun"="저글러\n조율가\n코디네이터\n재배열하는 사람\n멀티 씽커(Multi thinker)\n통제자\n협력자\n지휘자"}, {"Talent"="긍정", "Talent_eng"="Positivity", "Classify text"="R", "설명"="주변 사람들을 쉽게 사로잡는 긍정적인 열정을 가지고 있습니다. 이들은 낙관적이며 사람들로 하여금 자신들이 하려는 일에 열의를 갖게 만듭니다.", "성향"="낙관적이고 희망적이며 재미를 추구함", "행동 양상"="사기를 북돋는 밝은 정서적 환경을 조성함", "기여하는 것"="전염성이 강한 힘과 열정", "필요로 하는 것(요구 사항)"="삶의 기쁨과 극적인 순간을 경험할 자유", "좋아하는 것(가치)"="삶을 충만하게 영위", "싫어하는 것(가치)"="다른 사람을 기운 빠지게 하는 부정적인 사람들", "은유/이미지"="절반밖에 안 남은 유리잔이 아닌 절반이나 차있는 유리잔", "장벽(Barrier Label)"="너무 순진함", "adj"="재미있는\n낙관적인\n희망을 주는\n관대한\n들떠 있는\n행복한\n열광적인\n힘이 넘치는\n기쁨을 주는\n영향적이 있는\n호들갑스러운\n걱정이 없는\n긍정적인", "noun"="에너자이저\n낙관주의자\n격려자\n영향력을 미치는 사람\n코미디언\n예능인\n축하하는 사람\n인정하는 사람\n열렬한 지지자\n옹호자\n"}, {"Talent"="행동", "Talent_eng"="Activator", "Classify text"="I", "설명"="머리 속에 있는 생각을 행동으로 옮겨 실현시킬 수 있습니다. 이들은 말만 하기 보다는 당장 실행하기를 원합니다.", "성향"="아무것도 안 하는 상황을 참을 수 없음", "행동 양상"="추진력을 만들어냄", "기여하는 것"="긴박함을 불어넣음", "필요로 하는 것(요구 사항)"="토론은 적게, 행동은 많이", "좋아하는 것(가치)"="시작, 착수", "싫어하는 것(가치)"="기다림, 시간 낭비", "은유/이미지"="빠른 착수", "장벽(Barrier Label)"="두들겨보기도 전에 돌다리를 건넘", "adj"="참을성 없는\n영향력 있는\n행동 지향적인\n주도적인\n촉매제 역할을 하는\n추진력이 있는\n빠른", "noun"="촉매제\n주도적인 사람\n선동자\n착수자\n인플루엔서"}, {"Talent"="회고", "Talent_eng"="Context", "Classify text"="T", "설명"="과거에 대해서 생각하는 것을 즐깁니다. 이들은 과거에 대한 성찰을 통해서 현재를 이해합니다.", "성향"="조상을 감사히 여기고 과거 사건들을 중요하게 여김", "행동 양상"="중요한 역사를 기억함", "기여하는 것"="정확한 기억과 귀중한 수집품", "필요로 하는 것(요구 사항)"="논의를 진행하고 결정을 내리기 위한 관련 배경", "좋아하는 것(가치)"="회고", "싫어하는 것(가치)"="과거에 대한 망각", "은유/이미지"="백미러 - 안전 운전을 위한 필수 요소", "장벽(Barrier Label)"="과거에서 벗어나지 못함", "adj"="역사에 관심이 높은\n과거를 중시하는\n직관력이 있는\n강조하는\n수집을 즐기는\n학구적인", "noun"="역사가\n프레임제시자\n기록자\n고고학자\n족보학자"}, {"Talent"="공정성", "Talent_eng"="Consistency", "Classify text"="E", "설명"="사람들이 동등하게 취급되어야 한다는 점을 날카롭게 인식합니다. 이들은 모두가 따를 수 있는 안정적인 루틴과 명료한 규칙, 절차를 갈망합니다.", "성향"="개인이 무엇을 바라는지보다 그룹이 무엇을 필요로 하는지에 더 많은 관심을 가짐", "행동 양상"="차이를 줄이고 균일성을 높임", "기여하는 것"="예측 가능한 문화를 조성하는 규칙과 정책", "필요로 하는 것(요구 사항)"="표준적인 운영 절차", "좋아하는 것(가치)"="동일한 방식으로 무엇인가를 반복하는 것", "싫어하는 것(가치)"="불필요한 맞춤화", "은유/이미지"="대열을 맞춰 비행하는 한무리의 거위 떼", "장벽(Barrier Label)"="관계와 결과보다 규칙을 우선시함", "adj"="공정한\n똑같이 하는\n평등하게 대하는\n원칙적인\n예측 가능한\n일관성 있는\n정당한\n현실적인\n효율적인", "noun"="표준화하는 사람\n규칙 집행자\n체계를 만드는 사람\n심판"}, {"Talent"="존재감", "Talent_eng"="Significance", "Classify text"="I", "설명"="큰 영향을 미치기를 원합니다. 그들은 독립적이며, 프로젝트의 우선순위를 정할 때 그것이 조직이나 주위 사람들에게 얼마나 영향을 미칠지를 근거로 생각합니다.", "성향"="사람들에게 중요한 존재로 인식되어 중요한 일을 맡아 완수할 수 있는 기회에 관심이 있음", "행동 양상"="다른 사람들의 인식에서 영향을 받고 이를 통해 의욕을 냄", "기여하는 것"="더 많이 인정받고 싶어하는 마음", "필요로 하는 것(요구 사항)"="기량을 최대로 발휘할 의욕을 갖게 하고, 나의 진가를 알아봐 주는 사람들", "좋아하는 것(가치)"="성공한 사람들과의 교류", "싫어하는 것(가치)"="다른 사람들에게 존재감이 없거나 무시 당하는 것", "은유/이미지"="무대 중앙에 서거나 조명을 받는 것을 편하게 여기는 타고난 연예인", "장벽(Barrier Label)"="주목 받을 일만을 찾아 다님, 과시적임", "adj"="존경 받는\n믿을 수 있는\n성공적인\n눈에 띄는\n영향력이 있는\n원하는 것이 있는\n독립적인\n청중을 의식하는\n전문적인\n특출난", "noun"="손을 뻗는 사람\n예능인\n스타\n추구하는 사람\n열망하는 사람\n갈망하는 사람\n욕망하는 사람\n주장하는 사람"}, {"Talent"="미래지향", "Talent_eng"="Futuristic", "Classify text"="T", "설명"="미래와 가능성에서 영감을 얻습니다. 이들은 미래의 비전으로 사람들에게 영감을 줍니다.", "성향"="미래에 매료됨", "행동 양상"="앞으로 일어날 수 있는 일 또는 일어나야 하는 일을 예측하고 상상함", "기여하는 것"="미리 그려보기, 예상, 예측", "필요로 하는 것(요구 사항)"="예견되는 미래에 대해 말할 기회", "좋아하는 것(가치)"="미래를 생각하는 과정에서 얻는 영감", "싫어하는 것(가치)"="현재 상황에 만족하는 안일함", "은유/이미지"="비전", "장벽(Barrier Label)"="뜬구름 잡기", "adj"="창의적인\n영감을 주는\n상상력이 뛰어난\n상상력이 풍부한\n예상을 잘하는\n표현력이 뛰어난\n의사소통 능력이 있는\n직관력이 있는\n미래 지향적인", "noun"="예측가\n비전가\n꿈꾸는 사람\n앞을 내다보는 사람\n상상하는 사람\n예상하는 사람"}, {"Talent"="집중", "Talent_eng"="Focus", "Classify text"="E", "설명"="방향을 정해 일을 완수하며, 방향에서 벗어나지 않기 위해 필요한 수정을 해냅니다. 이들은 우선순위를 정한 다음, 실행합니다.", "성향"="굉장히 고지식하며 일부러 그런 태도를 고집함", "행동 양상"="목표에 도달할 때까지 인내함", "기여하는 것"="집중과 방향을 통한 명료함", "필요로 하는 것(요구 사항)"="우선순위를 설정할 수 있게 해주는 목표", "좋아하는 것(가치)"="끝을 염두에 둔 시작", "싫어하는 것(가치)"="잘못된 옆길로 새는 것", "은유/이미지"="무아지경", "장벽(Barrier Label)"="목적지에 도달하는 데 정신이 집중되어 있어 여정의 즐거움을 느끼지 못할 수 있음", "adj"="목표 지향적인\n끈기 있는\n의욕이 넘치는\n효율적인\n전념을 다하는\n진전을 중시하는\n선별적인\n집중을 방해하는 것을 피하는", "noun"="집중하는 사람\n우선순위를 정하는 사람\n방향을 잡는 사람\n목표를 설정하는 사람\n감독\n가이드"}, {"Talent"="주도력", "Talent_eng"="Command", "Classify text"="I", "설명"="존재감이 있습니다. 이들은 상황을 주도하고 의사결정을 내릴 수 있습니다.", "성향"="단도직입적이며 결단력이 있음", "행동 양상"="압력이 들어오면 저항함", "기여하는 것"="명확한 감정", "필요로 하는 것(요구 사항)"="도전과 갈등", "좋아하는 것(가치)"="통제를 벗어난 듯한 상황에서 통제력을 행사하는 것", "싫어하는 것(가치)"="소극적이고 회피하는 태도", "은유/이미지"="운전대를 잡고 있어야 편안함을 느낌", "장벽(Barrier Label)"="우두머리, 독재자", "adj"="결단력이 있는\n명확하게 하는\n의욕이 넘치는\n설득력 있는\n도전적인\n위압감을 주는\n단정적인\n통제적인\n자기 주장이 강한\n강요하는\n확고한\n솔직한", "noun"="통제가\n리더\n주도자\n명확하게 하는 사람\n설득자\n파이터\n도전자\n위압감을 주는 사람"}, {"Talent"="체계", "Talent_eng"="Discipline", "Classify text"="E", "설명"="정해진 절차와 구조를 즐깁니다. 스스로 만든 질서가 이들이 사는 세계를 가장 잘 설명해줍니다.", "성향"="제한된 자원을 효율적으로 관리함", "행동 양상"="미리 계획하고 그 다음에 계획을 따름", "기여하는 것"="정확성과 세부 지향", "필요로 하는 것(요구 사항)"="구조화되고 질서 있는 환경", "좋아하는 것(가치)"="질서 정연하게 정리된 것", "싫어하는 것(가치)"="혼란, 혼동, 감으로 일하는 것", "은유/이미지"="일렬로 줄지어가는 오리떼", "장벽(Barrier Label)"="변화에 저항할 수 있음", "adj"="예측 가능한\n세심한\n조직적인\n효율적인\n꼼꼼한\n구조적인\n깔끔한\n정돈된\n시기적절한\n예행연습을 하는\n계획적인\n정확한", "noun"="조직가\n계획가\n자율통제자\n설계자\n구성하는 사람\n완벽주의자"}, {"Talent"="화합", "Talent_eng"="Harmony", "Classify text"="R", "설명"="합의를 추구합니다. 이들은 갈등을 좋아하지 않고 갈등 대신 합의점을 찾고자 합니다.", "성향"="침착하고 평온함", "행동 양상"="감정적 에너지 소모를 없애려고 노력함", "기여하는 것"="평화와 사랑, 갈등을 피하는 접근법", "필요로 하는 것(요구 사항)"="합의점, 공통된 의견", "좋아하는 것(가치)"="그룹의 성과를 높이기 위해 개인적 주장을 희생함", "싫어하는 것(가치)"="갈등으로 인한 부정적 영향", "은유/이미지"="불편한 마음을 달램", "장벽(Barrier Label)"="갈등을 두려워함", "adj"="현실적인\n구체적인\n갈등을 줄이는\n협력적인\n선뜻 동의하는\n과업지향적인", "noun"="현실주의자\n실용주의자\n평화주의자\n협상가\n중재자\n대사\n외교관"}, {"Talent"="신념", "Talent_eng"="Belief", "Classify text"="E", "설명"="변하지 않는 확고한 핵심 가치를 가지고 있습니다. 이들의 삶의 목적은 이러한 가치에서 나옵니다.", "성향"="핵심 가치에 대한 열정이 있으며, 이를 타협하지 않음", "행동 양상"="중요한 일을 위해 기꺼이 희생함", "기여하는 것"="안정성, 명확성, 신념을 중시함", "필요로 하는 것(요구 사항)"="삶의 이유 또는 목적", "좋아하는 것(가치)"="이타심", "싫어하는 것(가치)"="신념에 맞지 않는 모든 것", "은유/이미지"="믿음을 전파하는 선교사", "장벽(Barrier Label)"="고집불통임", "adj"="확신이 있는\n안정적인\n변함없는\n지조있는\n열성적인\n헌신적인\n자기 희생적인", "noun"="선교사\n기여자\n믿는 사람\n이타주의자"}, {"Talent"="성취", "Talent_eng"="Achiever", "Classify text"="E", "설명"="에너지가 왕성하며 열심히 일합니다. 이들은 바쁘고 생산적인 데서 큰 만족감을 얻습니다.", "성향"="열심히 일함", "행동 양상"="업무 속도를 주도적으로 정함", "기여하는 것"="강도 높고 지치지 않는 노력", "필요로 하는 것(요구 사항)"="자신의 속도대로 일하는 재량권", "좋아하는 것(가치)"="업무 완수", "싫어하는 것(가치)"="성실하지 않은 태도", "은유/이미지"="경주 완주, 결승점 도착", "장벽(Barrier Label)"="사람보다 일을 더 중요하게 생각함", "adj"="의욕이 넘치는\n부지런한\n강렬한\n스스로 동기가 높은\n생산적인\n야심 있는\n독립적인", "noun"="수행자\n작업자\n생산자\n실행하는 사람\n마무리 짓는 사람\n완성가"}, {"Talent"="승부", "Talent_eng"="Competition", "Classify text"="I", "설명"="자신의 진전을 다른 사람의 성과와 비교해서 평가합니다. 이들은 1등을 차지하기 위해 분투하며 경쟁을 즐깁니다.", "성향"="경쟁자를 의식함", "행동 양상"="이기려고 노력함", "기여하는 것"="최고가 되려는 포부", "필요로 하는 것(요구 사항)"="비교 대상 및 동기부여가 되는 동료", "좋아하는 것(가치)"="최고의 자리에 있는 사람과 맞설 기회", "싫어하는 것(가치)"="2등을 하는 것", "은유/이미지"="아차상은 의미가 없으며 금메달만 인정함", "장벽(Barrier Label)"="패배를 인정하지 않음", "adj"="점수를 기록하는\n비교하는\n승리하는\n측정하는\n포부가 큰\n의욕이 넘치는\n강렬한\n선별적인", "noun"="승자\n점수 기록자\n비교하는 사람\n측정가"}, {"Talent"="심사숙고", "Talent_eng"="Deliberative", "Classify text"="E", "설명"="의사결정을 하거나 선택할 때 매우 신중합니다. 이들은 장애요소를 예측합니다.", "성향"="잠재적 위험을 관찰하는 데 경계를 늦추지 않음", "행동 양상"="잘못될 가능성이 있는 일을 예측함", "기여하는 것"="철저하고 성실한 접근", "필요로 하는 것(요구 사항)"="의견을 내기 전에 듣고 생각할 시간", "좋아하는 것(가치)"="리스크 직면 시 통제와 주의", "싫어하는 것(가치)"="성급한 판단", "은유/이미지"="유비무환, 평결에 앞서 숙고 과정을 거치는 배심원", "장벽(Barrier Label)"="망설임 - 아침에 일찍 일어나는 새가 벌레를 잡음에도 불구하고", "adj"="주의 깊은\n신중한\n보수적인\n분별 있는\n사려 깊은\n진지한\n비밀을 지키는\n관찰력이 있는\n방심하지 않는\n위험을 무릎쓰지 않는\n남에게 자기 얘기를 잘 안하는\n원칙을 따르는", "noun"="위험을 가늠하는 사람\n예방하는 사람\n수호자\n계획하는 사람"}, {"Talent"="사교성", "Talent_eng"="Woo", "Classify text"="I", "설명"="새로운 이들을 만나 그들의 마음을 얻는 일에 도전하기를 무척 즐깁니다. 이들은 어색한 분위기를 깨고 다른 사람과 인맥을 쌓는 데에서 만족감을 얻습니다.", "성향"="사람들과 금방 친해지고 외향적임", "행동 양상"="사람들과 교제할 때 주도권을 잡음", "기여하는 것"="사람들이 모이는 자리에 활기를 불어넣음", "필요로 하는 것(요구 사항)"="다양한 사람들과의 만남", "좋아하는 것(가치)"="처음 보는 사람과의 만남", "싫어하는 것(가치)"="정체되거나 위축된 인맥", "은유/이미지"="아이스 브레이킹 - 먼저 악수를 청함", "장벽(Barrier Label)"="겉치레를 중시하고 가벼움", "adj"="매력적인\n상호적인\n사회성이 강한\n영향력이 있는\n외향적인\n사교적인\n끌어들이는\n주도적인\n마음을 끄는\n사교적 에너지가 넘치는", "noun"="사교적인 사람\n매력적인 사람\n대화에 능한 사람\n접대자\n관계를 잘 맺는 사람\n먼저 시작하는 사람\n네트워커\n탐사자"}, {"Talent"="복구", "Talent_eng"="Restorative", "Classify text"="E", "설명"="문제를 능숙하게 다룹니다. 이들은 무엇이 잘못되었는지 파악하고 이를 해결하는 데 뛰어납니다.", "성향"="고충이나 문제가 발생해도 위축되지 않음", "행동 양상"="고충을 유발한 원인이나 장애를 일으키는 시스템 버그를 찾아 무엇이 문제인지 진단함", "기여하는 것"="문제 있는 상황에 대한 용기와 창의성", "필요로 하는 것(요구 사항)"="반드시 해결해야 하는 문제", "좋아하는 것(가치)"="해결책 찾기", "싫어하는 것(가치)"="무시하면 문제가 사라질 것이라는 생각", "은유/이미지"="탐정, 문제점 조사와 해결책 찾기", "장벽(Barrier Label)"="모든 상황에서 문제점을 찾는 경향이 있기 때문에 다른 사람에게 부정적으로 비추어짐", "adj"="문제에 주의를 기울이는\n의욕이 넘치는\n조사에 능한\n약점에 주의를 기울이는\n즉각 반응하는\n겁이 없는\n통찰력이 있는", "noun"="해결사\n진단자\n문제 해결자\n조사자\n회복시키는 사람\n소생시키는 사람"}]  # Basic info
        # "index는 나의 재능 테마 순서로. 0은 비워 놓음.\n나중에 테마 대조 정리할 때는 인덱스로 구분"
        "Basic info" <- w8
      }
      frame "data2" {
        w13 = string[][] [["1 가능성을 헤아리는 능력을 타고났습니다.", "3 현실을 헤아리는 능력을 타고났습니다."], ["1 다른 여러 경로를 고려합니다.", "25 단 하나의 목적지에 집중합니다."], ["2 관심이 가면 의지도 생깁니다.", "25 의지가 있어야 관심이 생깁니다."], ["2 항상 새로운 것을 배우는 데 관심이 있습니다.", "33 항상 새로운 사람을 만나는 데 관심이 있습니다."], ["3 머리를 따릅니다.", "5 가슴을 따릅니다."], ["3 진실은 객관적이며 측정할 수 있어야 합니다.", "16 진실은 정신적인 것이며 눈에 보이지 않을 수 있습니다."], ["4 성장과 배움을 위해 탐구하는 방식으로 접근함", "17 성장과 배움을 위해 습득하는 방식으로 접근함"], ["4 이해해야 할 개념에 대해 생각함", "34 해결해야 할 문제에 대해 생각함"], ["5 다른 사람의 기분을 잘 알아맞히는 편입니다.", "6 다른 사람의 성향을 잘 알아맞히는 편입니다."], ["5 직감에 따라 무엇을 해야 할지 결정합니다.", "3 데이터를 보고 무엇을 해야 할지 결정합니다."], ["6 당신이 누구인지 압니다.", "12 당신을 알고 싶고, 당신이 나를 알아주길 원합니다."], ["6 사람에서 출발해서 그 사람에게 적절한 일을 찾습니다.", "18 일에서 출발해서 그 일에 적절한 사람을 찾습니다."], ["7 제대로 못할 거라면 아예 시작도 하지 마십시오.", "20 아무것도 안 하는 것보다 뭐라도 하는 편이 낫습니다."], ["7 일을 제대로 하지 못하면 심한 죄책감이 듭니다.", "23 성공할 기회를 놓치면 너무나 후회가 됩니다."], ["8 적극적으로 개입하여 해결하기 위해 위험을 예측합니다.", "32 위험을 피하고 최소화하기 위해 위험을 예측합니다."], ["8 확신", "2 호기심"], ["9 외부에 있는 사람들을 수용하기 위해 노력합니다.", "28 내부에 있는 사람들의 합의를 도출하기 위해 노력합니다."], ["9 한 배에 탄 모든 사람을 차별없이 받아들입니다.", "10 배에 태울 사람을 선별적으로 선택합니다."], ["10 탁월함의 기준을 충족하거나 그 이상까지 달성하고 싶습니다.", "31 최고의 자리에 오르고 싶습니다."], ["10 훌륭한 성과를 쌓아가고 싶습니다.", "34 고장난 것을 고치고 싶습니다."], ["11 다른 사람들과 이야기할 때 생각이 잘 되고 가장 많이 배웁니다.", "4 혼자서 조용히 있을 때 생각이 잘 되고 가장 많이 배웁니다."], ["11 이야기를 하는 것은 사람들에게 나의 메시지를 이해시키는 데 도움이 됩니다.", "21 역사를 다시 이야기하는 것은 사람들이 과거를 기억하는 데 도움이 됩니다."], ["12 나는 사람들에게 투명하게 속을 드러내기 때문에 아는 친구들만 초대합니다.", "9 나는 사람들을 포용하는 성향이 있어 외부 사람들도 초대합니다."], ["12 이미 알고 있는 사람들에 대해 더 자세히 알고 싶습니다.", "33 더 많은 사람들을 알고 싶습니다."], ["13 타인의 성장을 알아차리고 촉진합니다.", "10 탁월함을 알아차리고 촉진합니다."], ["13 사람이 완성되게 하는 데 관심이 있습니다.", "30 일이 완수되게 하는 데 관심이 있습니다."], ["14 발견 가능성을 높이기 위해 마음의 창을 열어 둡니다.", "25 방해 가능성을 줄이기 위해 마음의 창을 닫아 둡니다."], ["14 경쟁 우위를 차지하려면 현실에서 벗어나 창의적으로 혁신하는 접근 방식이 가장 좋습니다.", "28 경쟁 우위를 차지하려면 현실적인 관점에서 효율적으로 협업하는 접근 방식이 가장 좋습니다."], ["15 매일매일이 다른 게 좋습니다.", "27 매일매일이 똑같은 게 좋습니다."], ["15 환경의 변화에 대응합니다.", "18 환경의 변화를 유도하거나 관리합니다."], ["16 신비를 인정합니다.", "3 진실을 입증합니다."], ["16 이미 존재하고 있으나 눈에는 보이지 않는 연결된 관계를 인식합니다.", "9 종종 발생하지만 눈에는 보이지 않는 사회적 배제를 인식합니다."], ["17 유용하게 사용될 수 있는 것들을 수집하기 좋아합니다.", "2 배우는 과정이 좋습니다."], ["17 실질적인 도구를 확보해 사람들과 공유함으로써 사람들을 돕습니다.", "14 창의적인 아이디어를 구상해 사람들과 공유함으로써 사람들을 돕습니다."], ["18 다양성", "25 단일성"], ["18 여러 개의 공을 공중에서 놀리는 저글링 곡예사", "7 하나의 공만 집요하게 쫓아가는 축구 선수"], ["19 근심이 없음", "3 진지함"], ["19 칭찬은 아무리 해도 지나치지 않습니다. 그래서 나는 칭찬에 후합니다.", "32 칭찬도 지나치면 해가 됩니다. 그래서 나는 칭찬에 인색합니다."], ["20 행동을 대신할 만한 것은 없습니다.", "4 사고를 대신할 만한 것은 없습니다."], ["20 제대로 이해할 때까지 계속 행동하십시오.", "32 제대로 이해할 때 행동으로 옮기십시오."], ["21 자연스럽게 과거의 일을 기억하고 가치를 부여합니다.", "24 자연스럽게 앞으로 일어날 수 있는 일 또는 일어나야 하는 일을 예측하고 상상합니다."], ["21 과거를 이해해야 앞으로 나아갈 수 있습니다.", "25 목표가 분명해야 앞으로 나아갈 수 있습니다."], ["22 사람들을 비슷하게 대우해야 공정성이 높아집니다.", "6 사람들을 다르게 대우해야 공정성이 높아집니다."], ["22 회전목마를 좋아합니다.", "15 롤러코스터를 좋아합니다."], ["23 존경받고 싶기 때문에 존경받을 만한 일을 해야 합니다.", "33 사람들을 내 편으로 만들고 싶기 때문에 매력을 키워야 합니다."], ["23 사람들이 나를 봐주고 나의 이야기를 들어주면 좋겠습니다.", "32 내가 사람들을 지켜보고 사람들의 이야기를 들었으면 좋겠습니다."], ["24 내일에 너무 몰두한 나머지 오늘을 맞을 준비가 되어 있지 않습니다.", "15 오늘에 너무 몰두한 나머지 내일을 맞을 준비가 되어 있지 않습니다."], ["24 더 나은 세상을 볼 수 있습니다.", "1 더 나은 세상으로 가는 길을 볼 수 있습니다."], ["25 내겐 목표가 있습니다.", "24 내겐 꿈이 있습니다."], ["25 달성하려고 계획하는 목표가 있습니다.", "27 목표 달성을 위한 계획이 있습니다."], ["26 대립을 통해 상황을 명쾌하게 정리합니다.", "28 화합을 통해 합의점을 찾습니다."], ["26 사람들이 당신에게 끌리는 이유는 당신의 생각을 알기 때문입니다.", "5 사람들이 당신에게 끌리는 이유는 당신이 사람들의 감정을 잘 헤아리기 때문입니다."], ["27 마감을 지키는 이유는 기분이 좋아지기 때문입니다.", "7 마감을 지키는 이유는 그래야 사람들이 나를 존중하기 때문입니다."], ["27 나무를 보느라 숲을 보지 못합니다.", "16 숲을 보느라 나무를 보지 못합니다."], ["28 가장 잘 풀리는 일을 합시다.", "29 가장 중요한 일을 하고 싶습니다."], ["28 나는 상호의존적인 사람이라 기꺼이 전문가의 의견을 따릅니다.", "8 나는 독립적인 사람이라 나 자신의 전문성에 자신있게 의존합니다."], ["29 옳은 길은 하나뿐이므로 다른 길에는 눈길을 주지 않을 것입니다.", "1 가능한 길은 많으므로 전부 고려해 봐야 합니다."], ["29 믿는 것을 봅니다.", "3 보는 것을 믿습니다."], ["30 일을 완수하고 싶습니다.", "20 일을 시작하고 싶습니다."], ["30 치열한 성실함", "4 치열한 사고"], ["31 나는 남들의 성과를 지켜볼 때 더 나은 성과를 냅니다.", "23 나는 남들이 나의 성과를 지켜볼 때 더 나은 성과를 냅니다."], ["31 성과를 측정하는 수단이 되어 승리를 입증하는 것은 득점판입니다.", "3 경험을 수치화하고 이론을 입증하는 것은 데이터입니다."], ["32 브레이크와 같이 일의 속도를 늦추는 경향이 있습니다.", "20 가속 페달과 같이 일의 속도를 높이는 경향이 있습니다."], ["32 교제를 할 때 신중을 기함", "33 교제를 할 때 경계없이 적극적임"], ["33 넓은 인맥을 쌓을 수 있습니다.", "12 깊이 있는 인간 관계를 맺을 수 있습니다."], ["33 다른 사람을 내 편으로 만듦", "31 다른 사람을 이김"], ["34 문제 해결사", "1 지도 제작자"], ["34 의도적으로 문제 영역으로 들어가 원래 상태로 복구합니다.", "19 의도적으로 문제 영역을 피해 나의 감정 상태를 유지합니다."]]  # Theme compare
        n3 = call "(SubVI) Theme combination data.vi"() -> ("Talent order CB"=→"Talent order CB":string[], "arr Description CB"=→"arr Description CB":string[])  [unwired: 1 in]
        "Theme compare" <- w13
      }
      frame "preset1" {
        w14 = u32 9868950 ("Background black")
        "Background black" <- w14
        "Background black deep" <- w14
        "img space" <- i16 1 ("img space")
        "contents deep title 3" <- T4 "기여하는 것" ("contents deep title 4")
        "contents deep title 4" <- T4 "필요로 하는 것\n(요구 사항)" ("contents deep title 5")
        "contents deep title 5" <- T4 "좋아하는 것\n(가치)" ("contents deep title 6")
        "contents deep title 6" <- T4 "싫어하는 것\n(가치)" ("contents deep title 7")
        "contents deep title 7" <- T4 "은유/이미지" ("contents deep title 8")
        "contents deep title 8" <- T4 "장벽\n(Barrier Label)" ("contents deep title 3")
        "contents deep title 2" <- T4 "행동 양상" ("contents deep title 2")
        "contents deep title 1" <- T4 "성향" ("contents deep title 1")
        "Background black comp" <- w14
        "comp space" <- u32 20
        "Background black CB" <- w14
      }
      frame "preset2" {
        n4 = control-ref of="adj 1"() -> (w32:refnum<vi>)
        n5 = control-ref of="adj 2"() -> (w33:refnum<vi>)
        n6 = control-ref of="adj 3"() -> (w34:refnum<vi>)
        n7 = control-ref of="adj 4"() -> (w35:refnum<vi>)
        n8 = control-ref of="adj 5"() -> (w36:refnum<vi>)
        n9 = control-ref of="adj 6"() -> (w37:refnum<vi>)
        n10 = control-ref of="adj 7"() -> (w38:refnum<vi>)
        n11 = control-ref of="adj 8"() -> (w39:refnum<vi>)
        n12 = control-ref of="adj 9"() -> (w40:refnum<vi>)
        n13 = control-ref of="adj 10"() -> (w41:refnum<vi>)
        n14 = control-ref of="adj 11"() -> (w42:refnum<vi>)
        n15 = control-ref of="adj 12"() -> (w43:refnum<vi>)
        n16 = control-ref of="adj 13"() -> (w44:refnum<vi>)
        n17 = control-ref of="adj 14"() -> (w47:refnum<vi>)
        n18 = Build Array(w32, w33, w34, w35, w36, w37, w38) -> (w45:refnum<vi>[])
        n19 = Build Array(w39, w40, w41, w42, w43, w44, w47) -> (w46:refnum<vi>[])
        n20 = Build Array (concatenate)(w45, w46) -> (w48:refnum<vi>[])
        "adj array" <- w48
        n21 = Index Array(array=w48) -> (element=w29:refnum<vi>)  [unwired: 1 in]
        n22 = property class="Str (strict)"(reference=w29) -> ("Size"=w30:T9, "Text.FontSize"=w31:u32)  [unwired: 1 in, 2 out]
        n23 = for {
          tunnel: w30 -> [w51]
          tunnel: w48 -> [w50] mode=indexing
          tunnel: w31 -> [w49]
          n24 = property class="Str (strict)"(reference=w50, "Size"=w51, "Text.FontSize"=w49) -> ()  [unwired: 1 in, 2 out]
        }
      }
      frame "preset3" {
        n25 = control-ref of="contents deep 1"() -> (w72:refnum<vi>)
        n26 = control-ref of="contents deep 2"() -> (w60:refnum<vi>)
        n27 = control-ref of="contents deep 3"() -> (w59:refnum<vi>)
        n28 = control-ref of="contents deep 4"() -> (w58:refnum<vi>)
        n29 = control-ref of="contents deep 5"() -> (w54:refnum<vi>)
        n30 = control-ref of="contents deep 6"() -> (w55:refnum<vi>)
        n31 = control-ref of="contents deep 7"() -> (w56:refnum<vi>)
        n32 = control-ref of="contents deep 8"() -> (w57:refnum<vi>)
        n33 = control-ref of="contents deep title 1"() -> (w74:refnum<vi>)
        n34 = control-ref of="contents deep title 2"() -> (w63:refnum<vi>)
        n35 = control-ref of="contents deep title 3"() -> (w62:refnum<vi>)
        n36 = control-ref of="contents deep title 4"() -> (w61:refnum<vi>)
        n37 = control-ref of="contents deep title 5"() -> (w64:refnum<vi>)
        n38 = control-ref of="contents deep title 6"() -> (w65:refnum<vi>)
        n39 = control-ref of="contents deep title 7"() -> (w66:refnum<vi>)
        n40 = control-ref of="contents deep title 8"() -> (w67:refnum<vi>)
        n41 = Build Array(w72, w60, w59, w58, w54, w55, w56, w57) -> (w73:refnum<vi>[])
        "contents deep arr" <- w73
        n42 = Build Array(w74, w63, w62, w61, w64, w65, w66, w67) -> (w75:refnum<vi>[])
        "contents deep title arr" <- w75
        n43 = property class="Str (strict)"(reference=w74) -> ("Size"=w69:T9, "Text.FontSize"=w68:u32)  [unwired: 1 in, 2 out]
        n44 = property class="Str (strict)"(reference=w72) -> ("Size"=w70:T9, "Text.FontSize"=w71:u32)  [unwired: 1 in, 2 out]
        n45 = for {
          tunnel: w69 -> [w81]
          tunnel: w68 -> [w80]
          tunnel: w75 -> [w79] mode=indexing
          n46 = property class="Str (strict)"(reference=w79, "Size"=w81, "Text.FontSize"=w80) -> ()  [unwired: 1 in, 2 out]
        }
        n47 = for {
          tunnel: w70 -> [w78]
          tunnel: w71 -> [w77]
          tunnel: w73 -> [w76] mode=indexing
          n48 = property class="Str (strict)"(reference=w76, "Size"=w78, "Text.FontSize"=w77) -> ()  [unwired: 1 in, 2 out]
        }
      }
      frame "preset4" {
        n49 = control-ref of="contents comp 1"() -> (w87:refnum<vi>)
        n50 = control-ref of="contents comp 2"() -> (w86:refnum<vi>)
        n51 = control-ref of="contents comp 3"() -> (w85:refnum<vi>)
        n52 = control-ref of="contents comp 4"() -> (w84:refnum<vi>)
        n53 = control-ref of="contents comp 5"() -> (w88:refnum<vi>)
        n54 = control-ref of="contents comp 6"() -> (w89:refnum<vi>)
        n55 = control-ref of="contents comp 7"() -> (w90:refnum<vi>)
        n56 = control-ref of="contents comp 8"() -> (w91:refnum<vi>)
        n57 = control-ref of="contents comp 9"() -> (w95:refnum<vi>)
        n58 = control-ref of="contents comp 10"() -> (w94:refnum<vi>)
        n59 = control-ref of="contents comp 11"() -> (w93:refnum<vi>)
        n60 = control-ref of="contents comp 12"() -> (w92:refnum<vi>)
        n61 = control-ref of="contents comp 13"() -> (w96:refnum<vi>)
        n62 = control-ref of="contents comp 14"() -> (w97:refnum<vi>)
        n63 = control-ref of="contents comp 15"() -> (w98:refnum<vi>)
        n64 = control-ref of="contents comp 16"() -> (w99:refnum<vi>)
        n65 = Build Array(w87, w86, w85, w84, w88, w89, w90, w91) -> (w100:refnum<vi>[])
        n66 = Build Array(w95, w94, w93, w92, w96, w97, w98, w99) -> (w101:refnum<vi>[])
        n67 = Build Array (concatenate)(w100, w101) -> (→"content comp arr":refnum<vi>[])
      }
      frame "make card" {
        # "공백 데이터 제거"
        n68 = local read "Basic info"() -> (w105:T3)
        n69 = for {
          tunnel: w105 -> [w113] mode=indexing
          tunnel: [w112] -> w111 mode=indexing
          n70 = Unbundle By Name(w113) -> ("Talent"=w112:string)
        }
        n71 = local read "Theme compare"() -> (w110:string[][])
        n72 = Split 1D Array(array=w105, index=1) -> (second subarray=w103:T3)  [unwired: 1 out]
        n73 = call "(SubVI) organize theme compare.vi"("Talent array"=w111, "Theme compare"=w110) -> ("organize theme compare"=w109:string[][])
        n74 = for {
          tunnel: w105 -> [w117] mode=indexing
          tunnel: w109 -> [w116] mode=indexing
          tunnel: ctrl_enum_adj."(interact)img pos size" ("Enum") -> [w115]
          tunnel: w103 -> [w114]
          i -> [w118]
          n75 = while {
            shift-right: [w124] -> _
            shift-left: w115 -> [w126]
            tunnel: w118 -> [w123]
            tunnel: w117 -> [w122]
            tunnel: w116 -> [w121]
            shift-right: [w119] -> _
            shift-left: w114 -> [w120]
            stop <- w125 stop-if-true
            n76 = case shown="\"(interact)capture img\"" w126 {
              tunnel: [FALSE FALSE FALSE FALSE FALSE FALSE FALSE FALSE FALSE FALSE FALSE FALSE FALSE FALSE FALSE w368] -> w125
              tunnel: [ctrl_enum_adj."(interact)edit title" ("Enum") ctrl_enum_adj."(interact)edit contents" ("Enum") ctrl_enum_adj."(interact)capture img" ("Enum") w188 ctrl_enum_adj."(deep)edit title" ("Enum") ctrl_enum_adj."(deep)edit contents" ("Enum") ctrl_enum_adj."(deep)capture img" ("Enum") ctrl_enum_adj."(comp)img pos size" ("Enum") ctrl_enum_adj."(comp)edit title" ("Enum") ctrl_enum_adj."(comp)edit contents" ("Enum") ctrl_enum_adj."(comp)capture img" ("Enum") ctrl_enum_adj."(CB)img pos size" ("Enum") ctrl_enum_adj."(CB)edit title" ("Enum") ctrl_enum_adj."(CB)edit contents" ("Enum") ctrl_enum_adj."(CB)capture img" ("Enum") ctrl_enum_adj."(CB)edit title" ("Enum")] -> w124
              tunnel: w123 -> [_ _ _ w199 _ _ _ w260 _ _ _ w317 _ _ _ _]
              tunnel: w122 -> [_ w149 w163 w198 _ w227 w243 w259 _ w291 _ w316 w329 w355 w364 w380]
              tunnel: w121 -> [_ _ _ _ _ _ _ _ _ _ w305 _ _ _ _ _]
              tunnel: w120 -> [w127 w147 w159 w182 w206 w226 w237 w254 w270 w290 w301 w311 w328 w351 w365 w369]
              tunnel: [w127 w147 w159 w182 w206 w226 w237 w254 w270 w290 w301 w311 w327 w351 w365 w376] -> w119
              frame "(interact)img pos size" {
                # "Relocate initial position of Front panal"
                n77 = control-ref of="Background"() -> (w140:refnum<vi>)
                n78 = property class="ColBox"(reference=w140) -> ("Left"=w134:i32, "Top"=w133:i32)  [unwired: 1 in, 2 out]
                n79 = local read "img space"() -> (w130:i16)
                n80 = property class="ColBox"(reference=w140) -> ("Width"=w137:u32, "Height"=w136:u32)  [unwired: 1 in, 2 out]
                n81 = Subtract(x=w134, y=w130) -> (x-y=w132:i32)
                n82 = Subtract(x=w133, y=w130) -> (x-y=w131:i32)
                n83 = Multiply(x=w130, y=i16 2) -> (x*y=w128:i16)
                n84 = Add(x=w128, y=w137) -> (x+y=w138:u32)
                n85 = Add(x=w128, y=w136) -> (x+y=w139:u32)
                n86 = control-ref of="Pane"() -> (w144:refnum<vi>)
                n87 = Bundle By Name(cluster=T8 {"Horizontal"=0, "Vertical"=0} ("Origin"), "Horizontal"=w132, "Vertical"=w131) -> (w142:T8)
                n88 = Bundle By Name(cluster=T5 {"left"=0, "top"=0, "right"=380, "bottom"=620} ("subset rect 2"), "right"=w138, "bottom"=w139) -> (w135:T5)
                n89 = local write "subset rect"(w135) -> ()
                n90 = property class="Pane"(reference=w144, "Origin"=w142) -> ()  [unwired: 1 in, 2 out]
              }
              frame "(interact)edit title", Default {
                n91 = Unbundle By Name(w149) -> ("Talent"=w154:string, "Talent_eng"=w155:string, "Classify text"=w157:string)
                n92 = local write "toggle data"("adj" ("toggle data")) -> ()
                n93 = call "(SubVI) Theme color.vi"("Classify text"=w157) -> ("Classify color"=w158:u32)
                n94 = Concatenate Strings(w154, "\n(" ("string"), w155, ")" ("string")) -> (w156:string)
                n95 = local write "Talent"(w156) -> ()
                n96 = local write "Classify text"(w157) -> ()
                n97 = local write "Classify color"(w158) -> ()
              }
              frame "(interact)edit contents" {
                n98 = local read "toggle data"() -> (w165:string)
                n99 = Unbundle By Name(w163) -> ("noun"=w162:string)
                n100 = Unbundle By Name(w163) -> ("adj"=w161:string)
                n101 = Equal?(x=w165, y="adj" ("string")) -> (x = y?=w166:bool)
                n102 = Select(t=w161, s=w166, f=w162) -> (s? t:f=w160:string)
                n103 = call "(SubVI) Split string.vi"("text"=w160) -> ("text array"=w171:string[])
                n104 = local read "adj array"() -> (w169:refnum<vi>[])
                n105 = Array Size(array=w171) -> (size(s)=w170:i32)
                n106 = for {
                  tunnel: w169 -> [w181] mode=indexing
                  tunnel: w170 -> [w178]
                  tunnel: w171 -> [w180]
                  i -> [w179]
                  n107 = Less?(x=w179, y=w178) -> (x < y?=w176:bool)
                  n108 = Index Array(array=w180, index=w179) -> (element=w177:string)
                  n109 = Select(t=w177, s=w176, f="_____________________") -> (s? t:f=w174:string)
                  n110 = Concatenate Strings("· " ("string"), w174) -> (w172:string)
                  n111 = property class="Str (strict)"(reference=w181, "Value"=w172) -> ()  [unwired: 1 in, 2 out]
                }
              }
              frame "(interact)capture img" {
                n112 = local read "toggle data"() -> (w186:string)
                n113 = vi-ref "CliftonStrengths.vi"() -> (w201:refnum<vi>)
                n114 = Unbundle By Name(w198) -> ("Talent"=w184:string)
                n115 = Number To Decimal String(number=w199) -> (decimal integer string=w196:string)  [unwired: 1 in]
                n116 = invoke class="VI" method="FP.Get Image"(reference=w201) -> ("image data"=w203:T10)  [unwired: 5 in, 5 out]
                n117 = local read "subset rect"() -> (w197:T5)
                n118 = Concatenate Strings("img\\theme interaction\\", w186, "\\" ("string"), w196, "_", w184, ".png") -> (w204:string)
                n119 = call <vilib>:"Get Image Subset.vi"("subset rect"=w197, "image data"=w203) -> ("image subset"=w202:T10)  [unwired: 4 in, 1 out]
                n120 = String To Path(string=w204) -> (path=w194:path)
                n121 = call <vilib>:"Write PNG File.vi"("image data"=w202, "path to PNG file"=w194) -> ()  [unwired: 8 in, 2 out]
                n122 = local read "toggle data"() -> (w192:string)
                n123 = flat-sequence {
                  tunnel: w188 -> [_]
                  frame #0 {
                    n124 = local write "toggle data"("noun" ("toggle data")) -> ()
                  }
                }
                n125 = Equal?(x="adj" ("string"), y=w192) -> (x = y?=w191:bool)
                n126 = Select(t=ctrl_enum_adj."(interact)edit contents" ("Enum"), s=w191, f=ctrl_enum_adj."(deep)img pos size" ("Enum")) -> (s? t:f=w188:T7)
              }
              frame "(deep)img pos size" {
                # "Relocate initial position of Front panal"
                n127 = control-ref of="Background deep"() -> (w219:refnum<vi>)
                n128 = property class="ColBox"(reference=w219) -> ("Left"=w213:i32, "Top"=w212:i32)  [unwired: 1 in, 2 out]
                n129 = local read "img space"() -> (w209:i16)
                n130 = property class="ColBox"(reference=w219) -> ("Width"=w216:u32, "Height"=w215:u32)  [unwired: 1 in, 2 out]
                n131 = Subtract(x=w213, y=w209) -> (x-y=w211:i32)
                n132 = Subtract(x=w212, y=w209) -> (x-y=w210:i32)
                n133 = Multiply(x=w209, y=i16 2) -> (x*y=w207:i16)
                n134 = Add(x=w207, y=w216) -> (x+y=w217:u32)
                n135 = Add(x=w207, y=w215) -> (x+y=w218:u32)
                n136 = control-ref of="Pane"() -> (w223:refnum<vi>)
                n137 = Bundle By Name(cluster=T8 {"Horizontal"=0, "Vertical"=0} ("Origin"), "Horizontal"=w211, "Vertical"=w210) -> (w221:T8)
                n138 = Bundle By Name(cluster=T5 {"left"=0, "top"=0, "right"=380, "bottom"=620} ("subset rect 2"), "right"=w217, "bottom"=w218) -> (w214:T5)
                n139 = local write "subset rect"(w214) -> ()
                n140 = property class="Pane"(reference=w223, "Origin"=w221) -> ()  [unwired: 1 in, 2 out]
              }
              frame "(deep)edit title" {
                n141 = Unbundle By Name(w227) -> ("Talent"=w232:string, "Talent_eng"=w233:string, "Classify text"=w235:string)
                n142 = call "(SubVI) Theme color.vi"("Classify text"=w235) -> ("Classify color"=w236:u32)
                n143 = Concatenate Strings(w232, "\n(" ("string"), w233, ")" ("string")) -> (w234:string)
                n144 = local write "Talent deep"(w234) -> ()
                n145 = local write "Classify text deep"(w235) -> ()
                n146 = local write "Classify color deep"(w236) -> ()
              }
              frame "(deep)edit contents" {
                n147 = Cluster To Array(cluster=w243) -> (array=w242:string[])
                n148 = local read "contents deep arr"() -> (w239:refnum<vi>[])
                n149 = Array Subset(array=w242, index=4, length=8) -> (w238:string[])
                n150 = Unbundle By Name(w243) -> ("Talent"=w247:string, "Talent_eng"=w246:string, "설명"=w245:string)
                n151 = for {
                  tunnel: w239 -> [w253] mode=indexing
                  tunnel: w238 -> [w252] mode=indexing
                  n152 = property class="Str (strict)"(reference=w253, "Value"=w252) -> ()  [unwired: 1 in, 2 out]
                }
                n153 = Concatenate Strings(w247, "(" ("string"), w246, ") 테마가 특히 강한 사람들은 " ("string"), w245) -> (w244:string)
                n154 = local write "summary deep"(w244) -> ()
              }
              frame "(deep)capture img" {
                n155 = vi-ref "CliftonStrengths.vi"() -> (w264:refnum<vi>)
                n156 = Unbundle By Name(w259) -> ("Talent"=w257:string)
                n157 = Number To Decimal String(number=w260) -> (decimal integer string=w267:string)  [unwired: 1 in]
                n158 = invoke class="VI" method="FP.Get Image"(reference=w264) -> ("image data"=w266:T10)  [unwired: 5 in, 5 out]
                n159 = local read "subset rect"() -> (w255:T5)
                n160 = Concatenate Strings("img\\theme deep understanding\\deep\\", w267, "_", w257, ".png") -> (w268:string)
                n161 = call <vilib>:"Get Image Subset.vi"("subset rect"=w255, "image data"=w266) -> ("image subset"=w265:T10)  [unwired: 4 in, 1 out]
                n162 = String To Path(string=w268) -> (path=w269:path)
                n163 = call <vilib>:"Write PNG File.vi"("image data"=w265, "path to PNG file"=w269) -> ()  [unwired: 8 in, 2 out]
              }
              frame "(comp)img pos size" {
                # "Relocate initial position of Front panal"
                n164 = control-ref of="Background comp"() -> (w283:refnum<vi>)
                n165 = property class="ColBox"(reference=w283) -> ("Left"=w277:i32, "Top"=w276:i32)  [unwired: 1 in, 2 out]
                n166 = local read "img space"() -> (w273:i16)
                n167 = property class="ColBox"(reference=w283) -> ("Width"=w280:u32, "Height"=w279:u32)  [unwired: 1 in, 2 out]
                n168 = Subtract(x=w277, y=w273) -> (x-y=w275:i32)
                n169 = Subtract(x=w276, y=w273) -> (x-y=w274:i32)
                n170 = Multiply(x=w273, y=i16 2) -> (x*y=w271:i16)
                n171 = Add(x=w271, y=w280) -> (x+y=w281:u32)
                n172 = Add(x=w271, y=w279) -> (x+y=w282:u32)
                n173 = control-ref of="Pane"() -> (w287:refnum<vi>)
                n174 = Bundle By Name(cluster=T8 {"Horizontal"=0, "Vertical"=0} ("Origin"), "Horizontal"=w275, "Vertical"=w274) -> (w285:T8)
                n175 = Bundle By Name(cluster=T5 {"left"=0, "top"=0, "right"=380, "bottom"=620} ("subset rect 2"), "right"=w281, "bottom"=w282) -> (w278:T5)
                n176 = local write "subset rect"(w278) -> ()
                n177 = property class="Pane"(reference=w287, "Origin"=w285) -> ()  [unwired: 1 in, 2 out]
              }
              frame "(comp)edit title" {
                n178 = Unbundle By Name(w291) -> ("Talent"=w296:string, "Talent_eng"=w297:string, "Classify text"=w299:string)
                n179 = call "(SubVI) Theme color.vi"("Classify text"=w299) -> ("Classify color"=w300:u32)
                n180 = Concatenate Strings(w296, "\n(" ("string"), w297, ")" ("string")) -> (w298:string)
                n181 = local write "Talent comp"(w298) -> ()
                n182 = local write "Classify text comp"(w299) -> ()
                n183 = local write "Classify color comp"(w300) -> ()
              }
              frame "(comp)edit contents" {
                n184 = local read "content comp arr"() -> (w304:refnum<vi>[])
                n185 = for {
                  tunnel: w305 -> [w310] mode=indexing
                  tunnel: w304 -> [w309] mode=indexing
                  tunnel: [w308] -> w303 mode=indexing
                  n186 = property class="Str (strict)"(reference=w309, "Value"=w310) -> (reference out=w308:refnum<vi>)  [unwired: 1 in, 1 out]
                }
                n187 = local read "comp space"() -> (w302:u32)
                n188 = call "(SubVI) Optimizing text height.vi"("comp space"=w302, "content comp arr"=w303) -> ()  [unwired: 1 in]
              }
              frame "(comp)capture img" {
                n189 = vi-ref "CliftonStrengths.vi"() -> (w321:refnum<vi>)
                n190 = Unbundle By Name(w316) -> ("Talent"=w314:string)
                n191 = Number To Decimal String(number=w317) -> (decimal integer string=w324:string)  [unwired: 1 in]
                n192 = invoke class="VI" method="FP.Get Image"(reference=w321) -> ("image data"=w323:T10)  [unwired: 5 in, 5 out]
                n193 = local read "subset rect"() -> (w312:T5)
                n194 = Concatenate Strings("img\\theme deep understanding\\compare\\", w324, "_", w314, ".png") -> (w325:string)
                n195 = call <vilib>:"Get Image Subset.vi"("subset rect"=w312, "image data"=w323) -> ("image subset"=w322:T10)  [unwired: 4 in, 1 out]
                n196 = String To Path(string=w325) -> (path=w326:path)
                n197 = call <vilib>:"Write PNG File.vi"("image data"=w322, "path to PNG file"=w326) -> ()  [unwired: 8 in, 2 out]
              }
              frame "(CB)img pos size" {
                # "자기 자신 제거"
                # "Relocate initial position of Front panal"
                n198 = control-ref of="Background CB"() -> (w343:refnum<vi>)
                n199 = property class="ColBox"(reference=w343) -> ("Left"=w337:i32, "Top"=w336:i32)  [unwired: 1 in, 2 out]
                n200 = local read "img space"() -> (w333:i16)
                n201 = property class="ColBox"(reference=w343) -> ("Width"=w340:u32, "Height"=w339:u32)  [unwired: 1 in, 2 out]
                n202 = Subtract(x=w337, y=w333) -> (x-y=w335:i32)
                n203 = Subtract(x=w336, y=w333) -> (x-y=w334:i32)
                n204 = Multiply(x=w333, y=i16 2) -> (x*y=w331:i16)
                n205 = Add(x=w331, y=w340) -> (x+y=w341:u32)
                n206 = Add(x=w331, y=w339) -> (x+y=w342:u32)
                n207 = control-ref of="Pane"() -> (w347:refnum<vi>)
                n208 = Bundle By Name(cluster=T8 {"Horizontal"=0, "Vertical"=0} ("Origin"), "Horizontal"=w335, "Vertical"=w334) -> (w345:T8)
                n209 = Bundle By Name(cluster=T5 {"left"=0, "top"=0, "right"=380, "bottom"=620} ("subset rect 2"), "right"=w341, "bottom"=w342) -> (w338:T5)
                n210 = local write "subset rect"(w338) -> ()
                n211 = property class="Pane"(reference=w347, "Origin"=w345) -> ()  [unwired: 1 in, 2 out]
                n212 = Search 1D Array(1D array=w328, element=w329) -> (index of element=w330:i32)  [unwired: 1 in]
                n213 = Delete From Array(array=w328, index=w330) -> (array with subset deleted=w327:T3)  [unwired: 1 in, 1 out]
              }
              frame "(CB)edit title" {
                # "첫 번째부터"
                n214 = control-ref of="Talent1 CB"() -> (w354:refnum<vi>)
                n215 = control-ref of="Talent2 CB"() -> (w353:refnum<vi>)
                n216 = Index Array(array=w351, index=0) -> (element=w352:T11)
                n217 = call "(SubVI) Title CB.vi"("Talent CB"=w354, "Basic info element"=w355) -> ()  [unwired: 1 in]
                n218 = call "(SubVI) Title CB.vi"("Talent CB"=w353, "Basic info element"=w352) -> ()  [unwired: 1 in]
              }
              frame "(CB)edit contents" {
                n219 = local read "arr Description CB"() -> (w362:string[])
                n220 = local read "Talent order CB"() -> (w361:string[])
                n221 = Index Array(array=w365) -> (element=w363:T11)  [unwired: 1 in]
                n222 = Unbundle By Name(w364) -> ("Talent"=w360:string)
                n223 = Unbundle By Name(w363) -> ("Talent"=w359:string)
                n224 = call "(SubVI) Extract description CB.vi"("Talent 2"=w359, "Talent 1"=w360, "Talent order CB"=w361, "arr Description CB"=w362) -> ("Description CB"=w358:string)
                n225 = local write "Description CB"(w358) -> ()
              }
              frame "(CB)capture img" {
                # "첫 번째 idx 부터 제거"
                n226 = Index Array(array=w369, index=0) -> (element=w372:T11)
                n227 = vi-ref "CliftonStrengths.vi"() -> (w383:refnum<vi>)
                n228 = Unbundle By Name(w372) -> ("Talent"=w371:string)
                n229 = Unbundle By Name(w380) -> ("Talent"=w374:string)
                n230 = invoke class="VI" method="FP.Get Image"(reference=w383) -> ("image data"=w385:T10)  [unwired: 5 in, 5 out]
                n231 = local read "subset rect"() -> (w377:T5)
                n232 = Concatenate Strings("img\\theme combination\\", w374, "_", w371, ".png") -> (w386:string)
                n233 = call <vilib>:"Get Image Subset.vi"("subset rect"=w377, "image data"=w385) -> ("image subset"=w384:T10)  [unwired: 4 in, 1 out]
                n234 = String To Path(string=w386) -> (path=w387:path)
                n235 = call <vilib>:"Write PNG File.vi"("image data"=w384, "path to PNG file"=w387) -> ()  [unwired: 8 in, 2 out]
                n236 = Array Size(array=w369) -> (size(s)=w370:i32)
                n237 = Equal To 0?(x=w370) -> (x = 0?=w368:bool)
                n238 = Delete From Array(array=w369, index=0) -> (array with subset deleted=w376:T3)  [unwired: 1 in, 1 out]
              }
            }
          }
        }
      }
    }
  }
  n239 = flat-sequence {
    tunnel: w1 -> [_]
    frame #0 {
      w393 = 0  # string length
      # "data analysis"
      n240 = local read "Theme compare"() -> (w390:string[][])
      n241 = Initialize Array(0, 35 ("dimension size")) -> (w397:i32[])
      n242 = for {
        tunnel: w390 -> [w423] mode=indexing
        shift-right: [w421] -> w396
        shift-left: w397 -> [w422]
        tunnel: [w420] -> w394 mode=indexing
        shift-right: [w418] -> _
        shift-left: w393 -> [w419]
        shift-right: [w414] -> w391
        shift-left: "" -> [w413]
        n243 = for {
          tunnel: w423 -> [w435] mode=indexing
          shift-right: [w430] -> w421
          shift-left: w422 -> [w433]
          tunnel: [w429] -> w420 mode=indexing
          shift-right: [w427] -> w418
          shift-left: w419 -> [w426]
          tunnel: [w425] -> w415 if=w424
          n244 = call <vilib>:"Space Constant.vi"() -> ("String"=w436:string)
          n245 = Search/Split String(string=w435, search string/char (-)=w436) -> (substring before match=w434:string, match + rest of string=w425:string)  [unwired: 1 in, 1 out]
          n246 = String Length(string=w425) -> (length=w428:i32)
          n247 = Decimal String To Number(string=w434) -> (number=w429:i32)  [unwired: 2 in, 1 out]
          n248 = Index Array(array=w433, index=w429) -> (element=w432:i32)
          n249 = Max & Min(x=w428, y=w426) -> (max(x,y)=w427:i32)  [unwired: 1 out]
          n250 = Increment(x=w432) -> (x+1=w431:i32)
          n251 = Not Equal?(x=w427, y=w426) -> (x != y?=w424:bool)
          n252 = Replace Array Subset(array=w433, new element=w431, index=w429) -> (w430:i32[])
        }
        n253 = Not Equal?(x=w415, y="") -> (x != y?=w416:bool)
        n254 = Select(t=w415, s=w416, f=w413) -> (s? t:f=w414:string)
      }
      "테마 대조 재능 index" <- w394
      "가장 길이가 긴 설명.\n화합" <- w391
      n255 = local read "Basic info"() -> (w389:T3)
      n256 = for {
        tunnel: w389 -> [w412] mode=indexing
        tunnel: [w411] -> w388 mode=indexing
        n257 = Unbundle By Name(w412) -> ("Talent"=w411:string)
      }
      n258 = while {
        shift-right: [w409] -> _
        shift-left: w396 -> [w410]
        tunnel: w388 -> [w406]
        tunnel: [w400] -> w395 mode=indexing
        stop <- w407 stop-if-true
        w408 = 0 ("new element/subarray")
        n259 = Array Max & Min(array=w410) -> (max value=w404:i32, max index (indices)=w405:i32)  [unwired: 2 out]
        n260 = Number To Decimal String(number=w404) -> (decimal integer string=w403:string)  [unwired: 1 in]
        n261 = Index Array(array=w406, index=w405) -> (element=w401:string)
        n262 = Replace Array Subset(array=w410, new element=w408, index=w405) -> (w409:i32[])
        n263 = Concatenate Strings(w403, "_" ("string"), w401) -> (w400:string)
        n264 = Equal?(x=w408, y=w404) -> (x = y?=w407:bool)
      }
      "테마대조 출현 횟수" <- w395
    }
  }
